vi "Dashboard Main.vi"() -> ()   [LabVIEW 2019]
uses:
  <vilib>/Rock Robotics/WPI/Solenoid/WPI_SolenoidValue.ctl
  <vilib>/Utility/miscctls.llb/LVRowAndColumnTypeDef.ctl
  <vilib>/event_ctls.llb/eventvkey.ctl
  <vilib>/Rock Robotics/Network Tables/NT Read Boolean.vi
  <vilib>/Rock Robotics/Network Tables/NT Write String Array.vi
  <vilib>/Rock Robotics/WPI/Dashboard/WPI_DashboardLogging Global.vi
  <vilib>/Rock Robotics/Network Tables/NT Write Boolean.vi
panel:
  out "Co-Pilot":string="Copilot:\n-LT(0.5 or higher): Intake stow/ deploy toggle\n-RX: Manual Turret Control\n-D-Pad Vertical: Manual Magazine\n-D-Pad Horizontal: Transverse\nMenu: Control panel Pneumatic toggle\nSelect: Elevator Brake\n-LX: Manual Climb Pivot\n-LY: Manual Climb Elevator\n-LB: Automatic climb balancing\n-RB: Toggle Auto_Targeting"
  out "Pilot":string="Pilot\n-LY: Drive Forward\n-RX: Drive Turn\n-Rumble if flywheel spun up and locked on & balls\n-LT(0.5 or more): Intake\n-RT(0.5 or more): Fire and Flywheel spin up\n-RB: control panel manual control \n-LB: Outtake"
  out "appended array":dbl[][](array[numeric])
  in  "TCP":refnum<k5>
  out "Robot IP":string="0.0.0.0"
  out "Image Message":string="Timeout in Camera Communications"
  in  "Dashboard Tab":T1(tab)=enum."Operation"
  in  "Select Auto":string(combo)="Select Autonomous ..."
  out "NT Connection":bool
  out "JS1 Z":dbl(slide) scale=-1.0..1.0 scale format="%#_2e"
  out "JS1 Graph":cluster{"X":dbl, "Y":dbl}[](graph)
  out "JS1 Buttons":T2
  out "JS2 Z":dbl(slide) scale=-1.0..1.0 scale format="%#_2e"
  out "JS2 Graph":cluster{"X":dbl, "Y":dbl}[](graph)
  out "JS2 Buttons":T2
  out "Mode":T3(ring)=enum."Disconnected"
  out "Right Camera Perf":cluster{"Bandwidth (Mbps)":dbl, "FPS":dbl}
  out "Camera Image Right":T4(plugin-control)
  in  "Rec Mode":enum32{"Stop", "Record", "Playback"}(radio)
  in  "Camera Name Right":string(combo)="No Camera Selection"
  in  "Camera Settings Right":T5={"Frame Rate"=15, "Compression"=30, "Size"=1, "DB Camera Config"=FALSE} {"Frame Rate" scale=1.0..30.0; "Compression" scale=100.0..-1.0; "Size" items=["640x480", "320x240", "160x120"]}
  in  "DB/String 9":string
  in  "DB/String 8":string
  in  "DB/String 7":string
  in  "DB/String 6":string
  in  "DB/String 5":string
  in  "DB/String 4":string
  in  "DB/String 3":string
  in  "DB/String 2":string
  in  "DB/String 1":string
  in  "DB/String 0":string
  in  "DB/Slider 0":dbl(slide) scale=0.0..5.0
  in  "DB/Slider 1":dbl(slide) scale=0.0..5.0
  in  "DB/Slider 2":dbl(slide) scale=0.0..5.0
  in  "DB/Slider 3":dbl(slide) scale=0.0..5.0
  out "DB/LED 3":bool
  out "DB/LED 2":bool
  out "DB/LED 1":bool
  out "DB/LED 0":bool
  in  "DB/Button 3":bool
  in  "DB/Button 2":bool
  in  "DB/Button 1":bool
  in  "DB/Button 0":bool caption="New Name"
  in  "Test Slider":dbl(slide) scale=0.0..100.0 scale format="%#_3g"
  in  "On/Off":bool caption="Solenoid"
  in  "Test Name":u16(ring) items=["Select the test to run..."]
  in  "Test Tree":string(tree)
  in  "Motor":cluster{"Value":dbl, "Enable":bool} {"Value" scale=-1.0..1.0 scale format="%#_3g"}
  out "Progress":T6 {"Test Progress" scale=0.0..100.0}
  in  "Rev/Fwd":cluster{"Forward":bool, "Reverse":bool}
  in  "Test Ring":u16(ring) items=["Monochrome", "Color"]
  out "Cmd Status":string
  in  "Execute Command":bool
  in  "Command Params":string[][](table)
  in  "Command Selection":i32(listbox)
  in  "CheckList":i32(listbox)
  in  "Color_Sensor_Values":enum32{"Page 1"}(tab)
  out "Match_Confidence":dbl
  out "Current_B":dbl
  out "Current_G":dbl
  out "Current_R":dbl
  out "Matched_Color_Name":string="No_Value"
  out "Control_Panel":enum32{"Controls"}(tab)
  in  "time_to_run":dbl
  in  "Spinwheel_Throttle":dbl
  in  "Red_B":dbl
  in  "Red_G":dbl
  in  "Red_R":dbl
  in  "Yellow_R":dbl
  in  "Yellow_G":dbl
  in  "Yellow_B":dbl
  in  "Blue_B":dbl
  in  "Blue_G":dbl
  in  "Blue_R":dbl
  in  "Green_R":dbl
  in  "Green_G":dbl
  in  "Green_B":dbl
  out "Magazine":enum32{"Controls"}(tab)
  in  "Max_Magazine_Speed":dbl=1050.0
  in  "Unjam_Speed":dbl
  in  "Firing_Speed":dbl=1.0
  in  "Loading_Speed":dbl=1.0
  in  "Bottom_IR_Theshold":dbl=1.0
  in  "Bottom_Middle_IR_Threshold":dbl=1.5
  in  "Top_Middle_IR_Threshold":dbl=2.0
  in  "Top_IR_Threshold":dbl=1.0
  out "Drive":enum32{"Controls"}(tab)
  in  "Drive_IMU_Yaw":dbl
  in  "Left_P":dbl=1.0
  in  "Left_I":dbl
  in  "Left_D":dbl
  in  "Left_F":dbl
  in  "Right_P":dbl=1.0
  in  "Right_I":dbl
  in  "Right_D":dbl
  in  "Right_F":dbl
  out "Flywheel":enum32{"Controls"}(tab)
  in  "Flywheel_F":dbl=0.0001
  in  "Flywheel_D":dbl
  in  "Flywheel_I":dbl
  in  "Flywheel_P":dbl=0.0001
  out "Turret":enum32{"Controls"}(tab)
  in  "Turret_D":dbl
  in  "Turret_I":dbl=1e-05
  in  "Turret_P":dbl=0.05
  in  "Turret_Upper_Limit":dbl=65.0
  in  "Turret_Lower_Limit":dbl=-90.0
  out "Climb":enum32{"Controls"}(tab)
  out "Intake":enum32{"Controls"}(tab)
  in  "Intake_Speed":dbl=0.7
  in  "extend_delay(ms)":dbl=1000.0
  in  "retract_delay(ms)":dbl=1000.0
  in  "Hopper Input":T7=enum."Reverse"
  in  "Intake Input":T7=enum."Reverse"
  out "No-Op Signal From Robot":bool
  out "Bottom_Middle_IR":bool
  out "Flywheel_Spun_Up":bool
  in  "Auto Selector":string(combo)="No-Op"
  out "Top_IR":bool
  out "Bottom_IR":bool
  out "Top_Middle_IR":bool
  out "Drive_IMU_Yaw":dbl
  out "Climb_IMU_Yaw":dbl
  out "Turret_Relative_Position":dbl
  out "Climb_Bottom_Limit":bool
  out "Climb_Top_Limit":bool
  out "Zero_Turret_Spin":bool
  out "Elevator_Right_Position(Native)":dbl
  out "Elevator_Left_Position(Native)":dbl
  out "Climb_Pivot_Position":dbl
  out "Right_Drive_Position":dbl
  out "Left_Drive_Position":dbl
  out "Control_Panel_Velocity(RPM)":dbl
  out "Control_Panel_Position":dbl
  out "Turret_Velocity(RPM)":dbl
  out "Turret_Absolute_Position":dbl
  out "Magazine_Velocity(RPM)":dbl
  out "Magazine_Position":dbl
  out "Flywheel_Right_Velocity":dbl
  out "Flywheel_Left_Velocity":dbl
  out "Right_Drive_Velocity(RPM)":dbl
  out "Left_Drive_Velocity(RPM)":dbl
  out "Climbing Active":bool
  out "Targetting_Active":bool
  out "Ball Serialized":bool
  out "Match Color Game Data (Stage 3)":string="No_Value"
  out "Camera Image":T4(plugin-control)
  in  "Camera Name":string(combo)="No Camera Selection"
  in  "Camera Settings":T5={"Frame Rate"=15, "Compression"=30, "Size"=1, "DB Camera Config"=FALSE} {"Frame Rate" scale=1.0..30.0; "Compression" scale=100.0..-1.0; "Size" items=["640x480", "320x240", "160x120"]}
  out "Camera Perf":string="                          "
  out "Tree":string(tree)
  out "Background":bool
  # "Joysticks"
  # "Drive Motors"
  # "Front"
  # "Right"
  # "Left"
  # "Back"
  # "HW"
  # "This tab is a great place for autonomous settings and robot-specific values.\nPlace controls and indicators inside this tab and match name to\nDashboard Variables on robot. You can also delete this comment."
  # "HW"
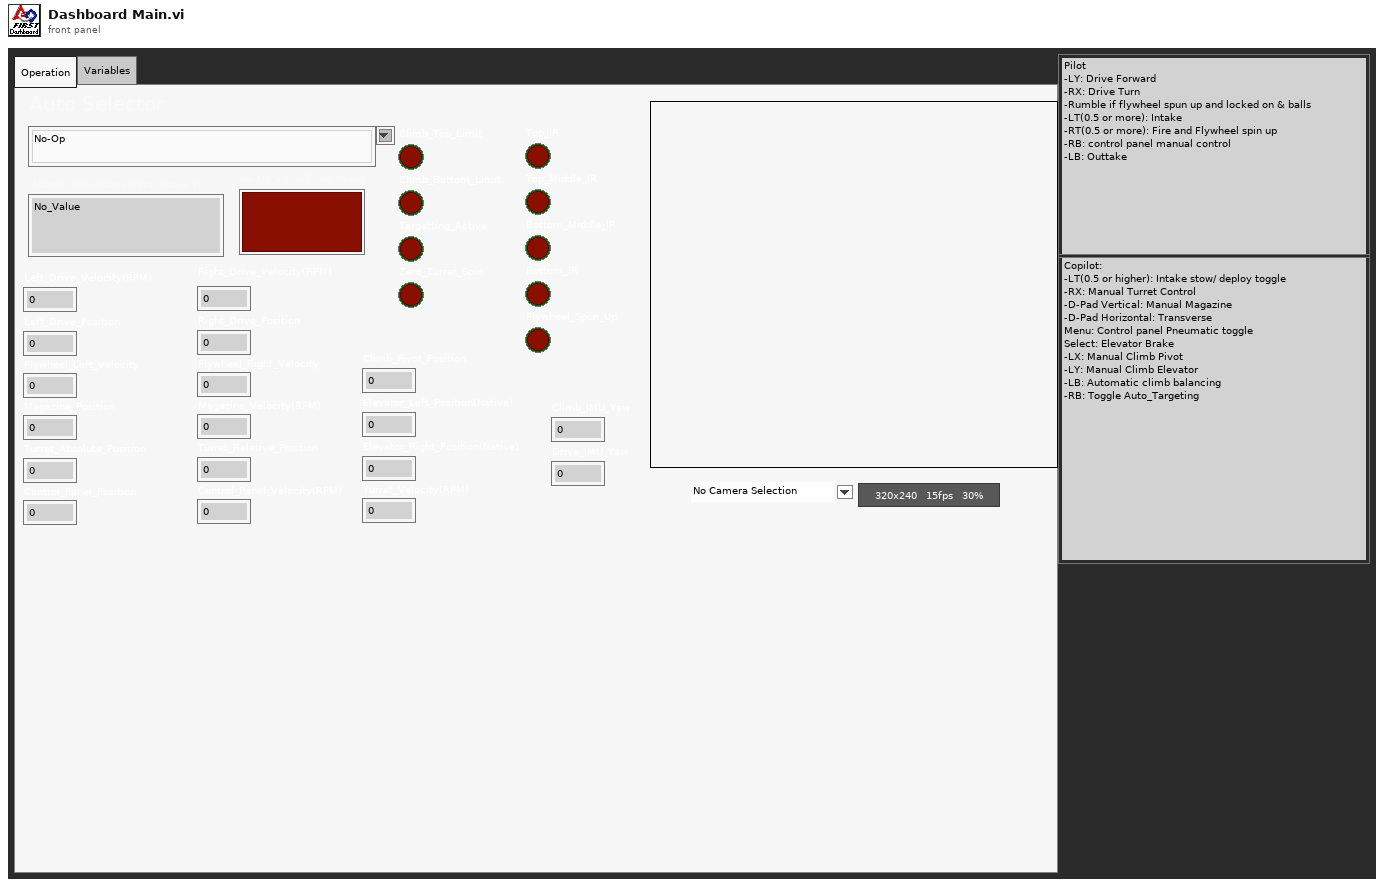
[diagram p1: front panel]
types:
  T1 = enum32{"Drive", "Camera", "Basic", "Custom", "Test", "Commands", "Checklist", "Calibration", "Operation", "Auto", "Variables"}
  T2 = cluster{bool, bool, bool, bool, bool, bool, bool, bool, bool, bool, bool, bool}
  T3 = enum8{"Tele-Op Disabled", "Tele-Op Enabled", "Auto Disabled", "Auto Enabled", "Test Disabled", "Test Enabled", "Disconnected", "No Code", "E-Stop"}
  T4 = typedef "IMAQ Image.ctl" = refnum<image>
  T5 = cluster{"Frame Rate":i32, "Compression":i32, "Size":u16, "DB Camera Config":bool}
  T6 = cluster{"Test Progress":u8, "Test Progress Text":string}
  T7 = typedef "WPI_SolenoidValue.ctl" = enum16{"Off", "On", "Forward", "Reverse"}
  T8 = cluster{"Save Path":path, "Interval (s)":dbl, "Keep":i32}
  T9 = enum32{"Drive", "Camera", "Basic", "Custom", "Test", "Commands", "Checklist", "Variables"}
  T10 = typedef "Image Type" = u32
  T11 = cluster{"IDs":cluster{"RPC field ID":u16, "Unique ID":u16}, "String":string}
  T12 = cluster{"Camera Image":refnum<vi>, "Dashboard Tab":refnum<vi>, "Background":refnum<vi>, "Rec Mode":refnum<vi>, "Test Slider":refnum<vi>, "On/Off ":refnum<vi>, "Test Ring":refnum<vi>, "Rev/Fwd":refnum<vi>, "Test Name":refnum<vi>, "Motor":refnum<vi>, "Progress":refnum<vi>, "CheckList":refnum<vi>, "Tree":refnum<vi>, "Test Tree":refnum<vi>, "Command Params":refnum<vi>, "Command Selection":refnum<vi>, "Execute Command":refnum<vi>, "Cmd Status":refnum<vi>, "Camera Settings":refnum<vi>, "Camera Name":refnum<vi>, "Camera Perf":refnum<vi>, "Camera Settings Right":refnum<vi>, "Camera Name Right":refnum<vi>, "Camera Image Right":refnum<vi>}
  T13 = cluster{"Error Strings":string, "Disable Counts":cluster{u16, u16}, "Rail Faults":cluster{u16, u16, u16}, "Robot IP":string, "DB Mode":u8, "Event Info":cluster{"Name":string, "Type":u8, "Number":u16, "Replay":u8}}
  T14 = cluster{"Storage":cluster{"Disk Free":u64, "RAM Block":u32, "RAM free":u32}, "CPU Utilization":cluster{"CPU % ISR":sgl, "CPU % Time Crit":sgl, "CPU % Timed Str":sgl, "CPU % High":sgl, "CPU % Above":sgl, "CPU % Normal":sgl, "CPU % Low":sgl}, "CAN":cluster{"% Bus Utilization":sgl, "Bus Off Cnt":u32, "TX_FIFO Full Cnt":u32, "Receive Error Cnt":u8, "Transmit Error Cnt":u8}, "HID":cluster{"HID Outputs":u32, "Rumble Low":u16, "Rumble High":u16}[]}
  T15 = cluster{"Status bits":cluster{"Test Mode":bool, "Autonomous":bool, "Enabled":bool, "Code Start":bool, "Brownout":bool, "Reserved 2":bool, "Reserved 3":bool, "E-Stop":bool}, "Code Trace":cluster{"Disabled":bool, "TeleOp":bool, "Auto":bool, "Test":bool}, "Controller Type":enum16{"unknown", "cRIO", "roboRio"}, "Code?":enum16{"unknown", "noCode", "code"}, "Battery V":dbl}
  T16 = cluster{"Control Bits":cluster{"TestMode":bool, "Autonomous":bool, "Enabled":bool, "FMS Present":bool, bool, bool, bool, "E-Stop":bool}, "Team Station ":u8, "Countdown":sgl, "Joystick Values":cluster{"Axes":dbl[], "Buttons":bool[], "POVs":i16[]}[]}
  T17 = cluster{"Axes":dbl[], "Buttons":bool[], "POVs":i16[]}[]
  T18 = cluster{"Axes":dbl[], "Buttons":bool[], "POVs":i16[]}
  T19 = cluster{"Buttons[0]":bool, "Buttons[1]":bool, "Buttons[2]":bool, "Buttons[3]":bool, "Buttons[4]":bool, "Buttons[5]":bool, "Buttons[6]":bool, "Buttons[7]":bool, "Buttons[8]":bool, "Buttons[9]":bool, "Buttons[10]":bool, "Buttons[11]":bool}
  T20 = cluster{"Global Rectangle":i32[], "Contours":cluster{"Contour Type":u32, "ROI Type":u32, "Points":i32[]}[]}
  T21 = cluster{"Camera Name":string, string, "Saved DB Images Info":cluster{"Save Path":path, "Interval (s)":dbl, "Keep":i32}}
  T22 = cluster{"Camera Name Right":string, string, "Saved DB Images Info":cluster{"Save Path":path, "Interval (s)":dbl, "Keep":i32}}
  T23 = cluster{"Operation":enum16{"Update", "Clear"}, "Color Box":u32}[]
  T24 = typedef "eventvkey.ctl" = enum16{"ASCII", "Enter", "Return", "Shift", "Ctrl", "Alt", "Cmd", "Opt", "Caps", "NumLock", "Clear", "Break", "Up", "Down", "Left", "Right", "Insert", "Delete", "Home", "End", "PageUp", "PageDown", "Escape", "Help", "Pause", "ScrollLock", "F1", "F2", "F3", "F4", "F5", "F6", "F7", "F8", "F9", "F10", "F11", "F12", "F13", "F14", "F15", "F16", "F17", "F18", "F19", "F20", "F21", "F22", "F23", "F24", "Play", "VolumeUp", "VolumeDown", "Mute", "Two Byte Char"}
  T25 = cluster{"Image Size":bool, "Image Type":bool, "Pixel Value":bool, "ROI Information":bool, "Zoom Factor":bool}
  T26 = cluster{"Operation":enum16{"Update", "Clear"}, "Color Box":u32}
  T27 = typedef "LVRowAndColumnTypeDef.ctl" = cluster{"Row":i32, "Column":i32}
  T28 = cluster{"Shift":bool, "Ctrl":bool, "Alt":bool, "Cmd":bool, "Opt":bool}
  T29 = enum32{"Drive", "Camera", "Basic", "Custom", "Test", "Commands", "Checklist", "Variables", "Calibration"}
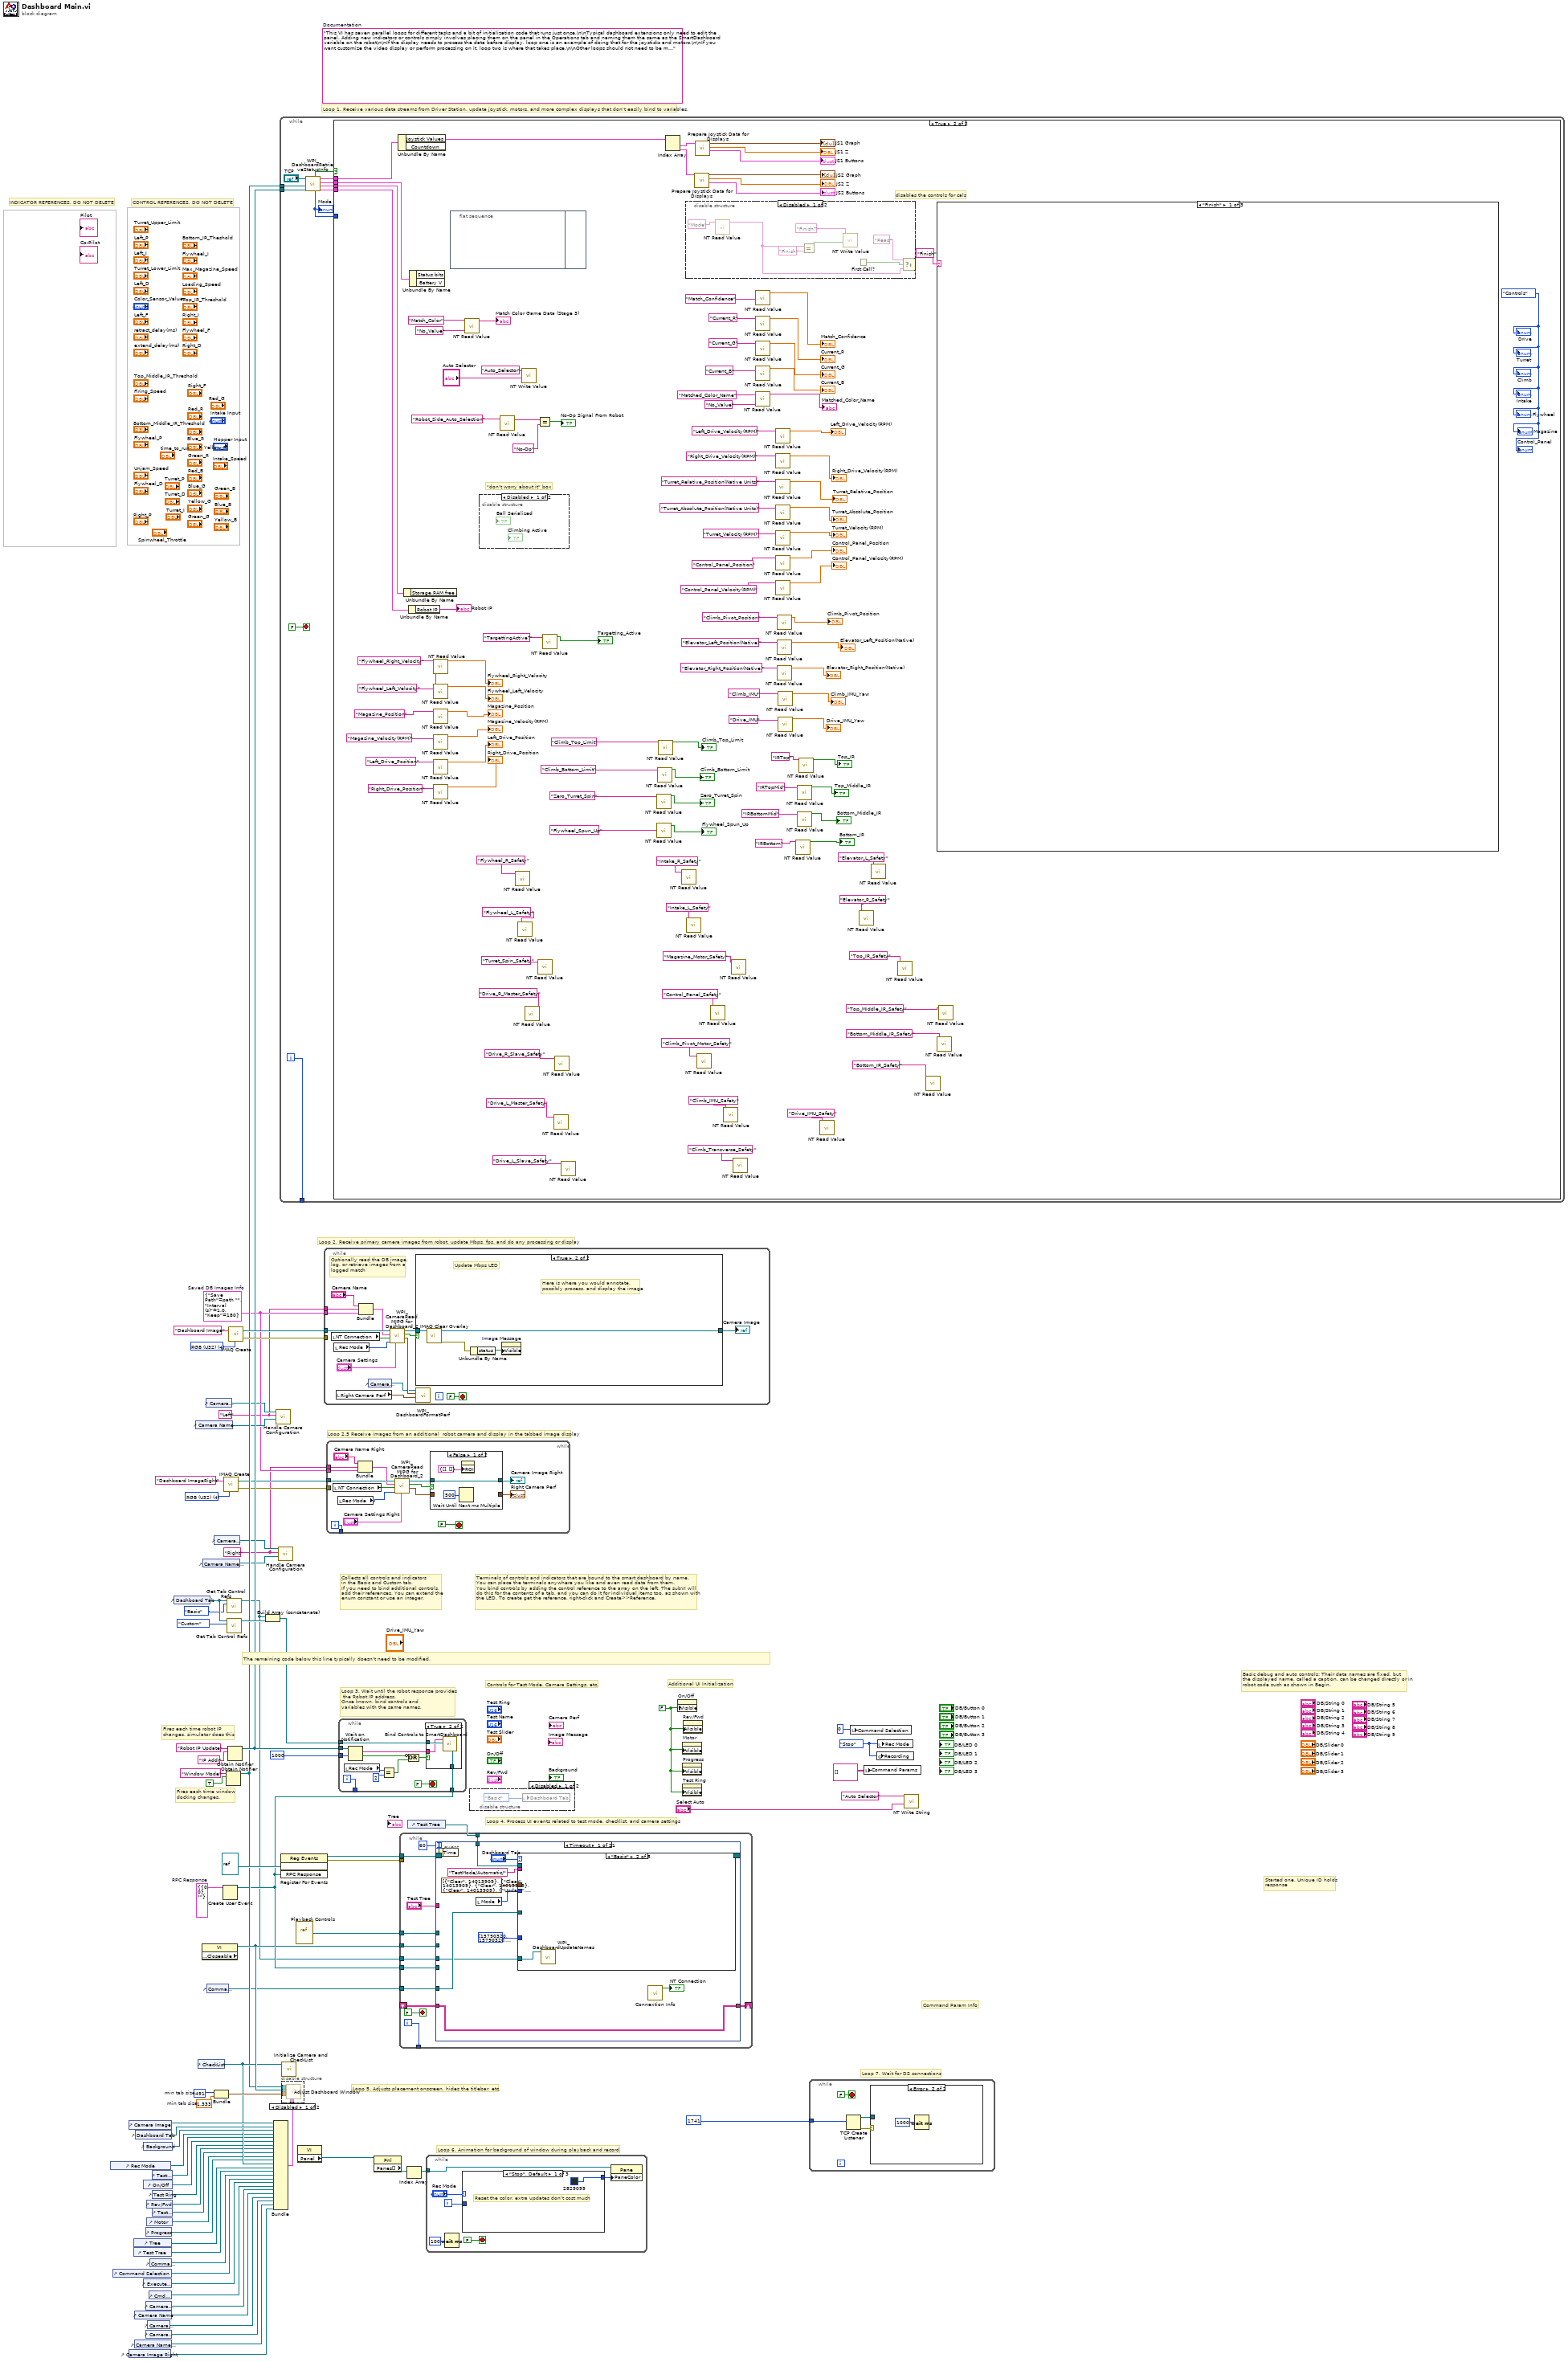
[diagram p0: block diagram]
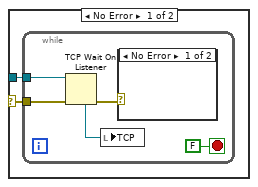
[diagram p5: hidden frame]
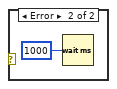
[diagram p6: hidden frame]
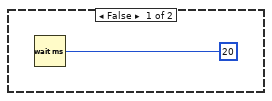
[diagram p7: hidden frame]
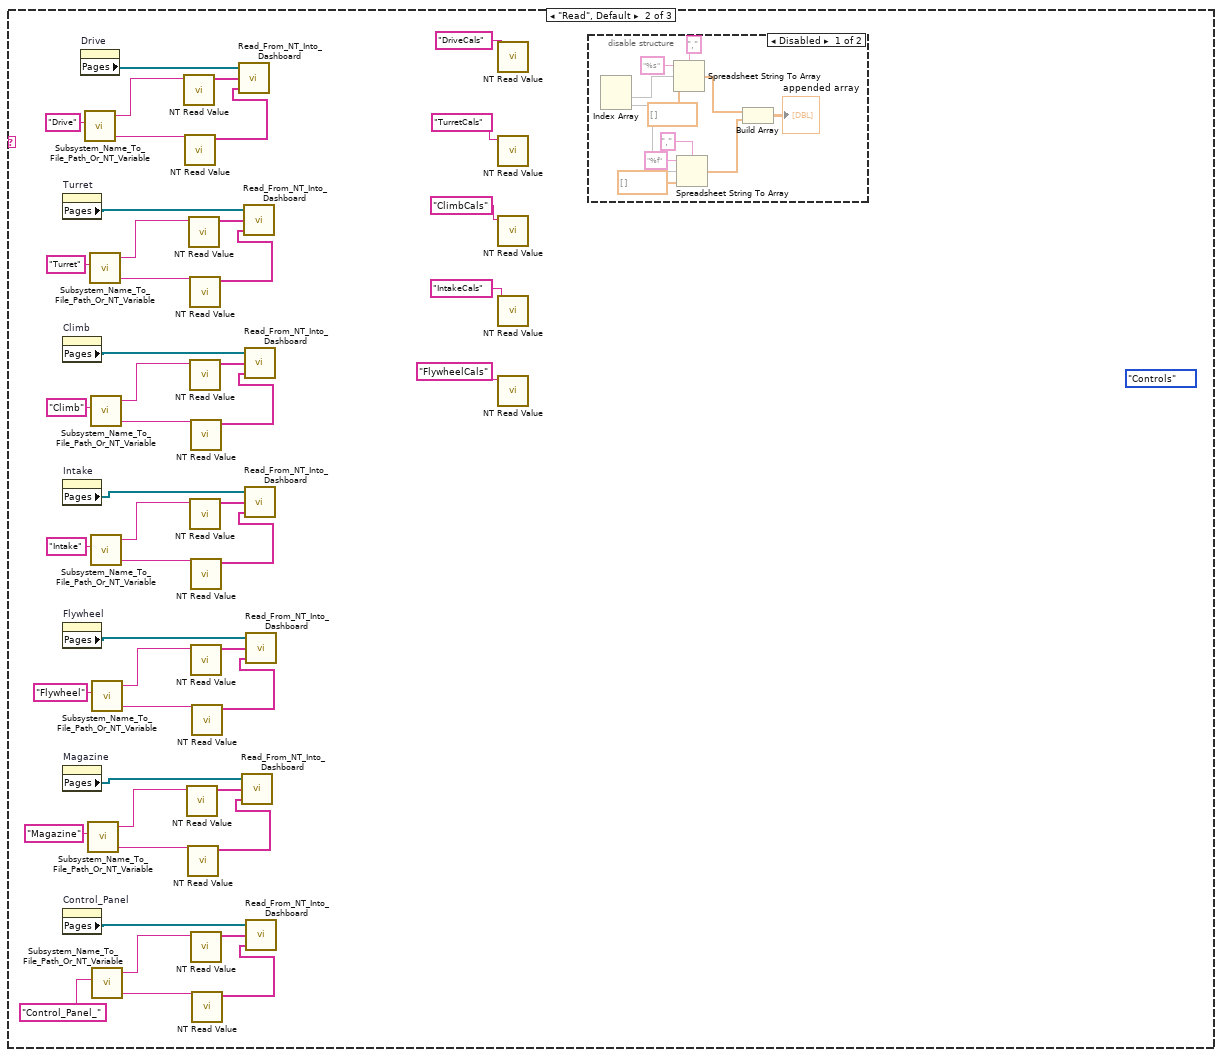
[diagram p10: hidden frame]
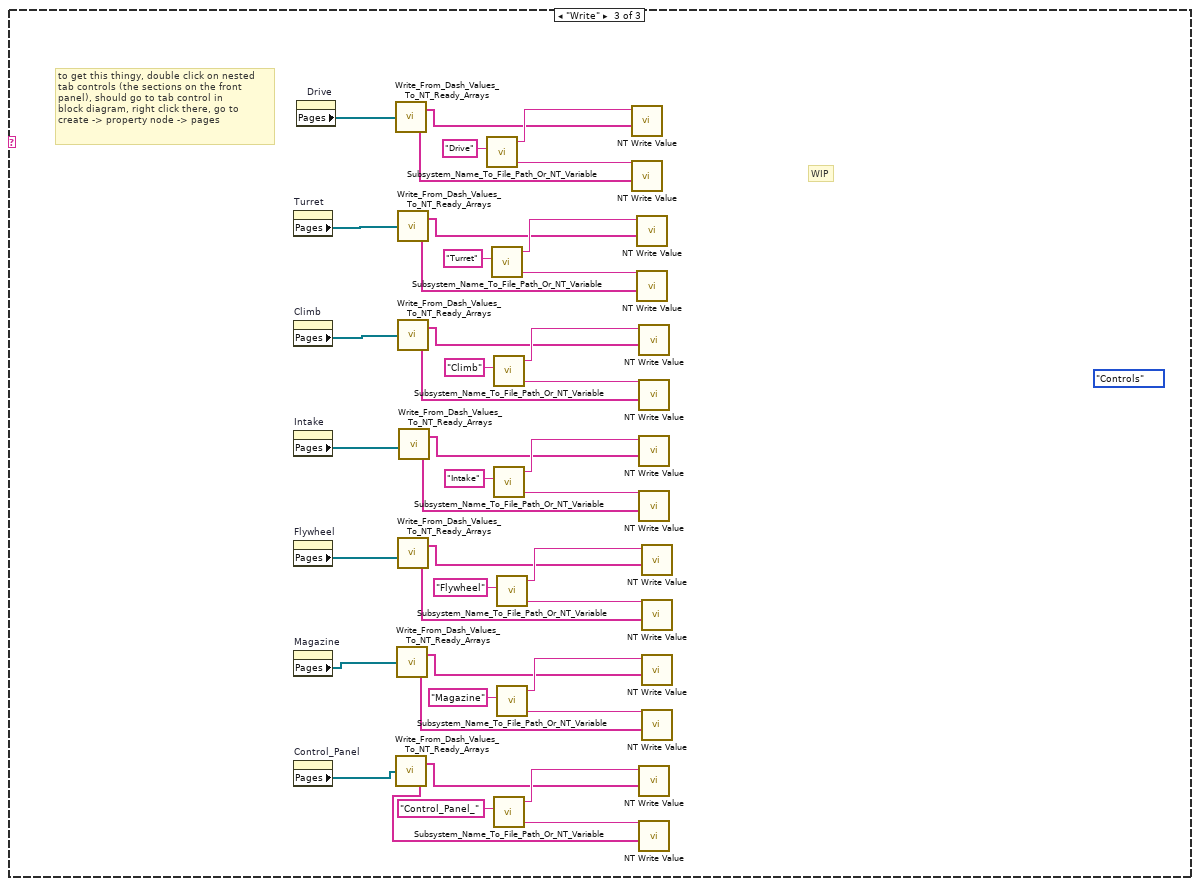
[diagram p12: hidden frame]
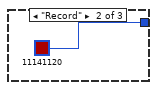
[diagram p13: hidden frame]
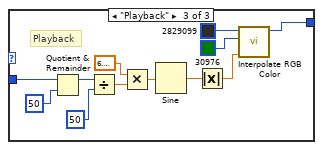
[diagram p14: hidden frame]
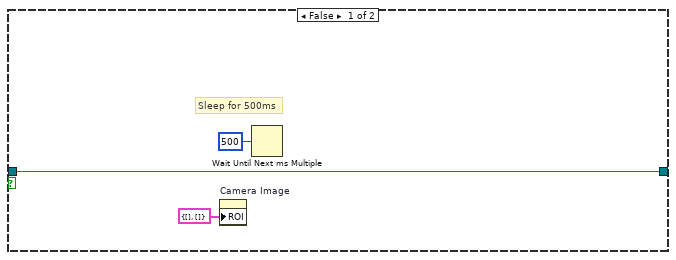
[diagram p16: hidden frame]
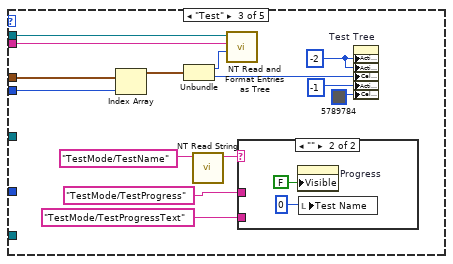
[diagram p18: hidden frame]
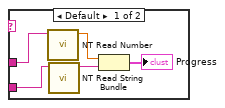
[diagram p19: hidden frame]
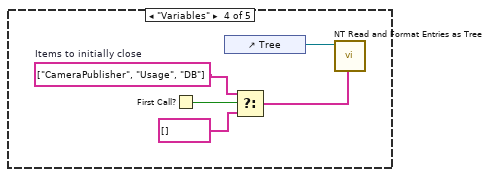
[diagram p20: hidden frame]
diagram:
  w3 = T8 {"Save Path"=path "", "Interval (s)"=1.0, "Keep"=180}  # Saved DB Images Info
  w2 = "Right"
  w1 = "Left"
  w13 = T10 4 items=["Grayscale (U8)", "Grayscale (I16)", "Grayscale (SGL)", "Complex (CSG)", "RGB (U32)", "HSL (U32)", "RGB (U64)"] ("Image Type")
  w29 = T11 {"IDs"={"RPC field ID"=0, "Unique ID"=0}, "String"=""}  # RPC Response
  w51 = 491  # min tab size
  w50 = 1.333  # min tab size
  w58 = enum32{"Stop", "Record", "Playback"}."Stop" ("Rec Mode")
  w35 = FALSE ("Visible")
  (unwired) "This VI has seven parallel loops for different tasks and a bit of initialization code that runs just once.\n\nTypical dashboard extensions only need to edit the panel. Adding new indicators or controls simply involves placing them on the panel in the Operations tab and naming them the same as the SmartDashboard variable on the robot\n\nIf the display needs to process the data before display, loop one is an example of doing that for the joysticks and motors.\n\nIf you want customize the video display or perform processing on it, loop two is where that takes place.\n\nOther loops should not need to be modified. They are pretty standard, and document the task they perform."  # Documentation
  w75 = T10 4 items=["Grayscale (U8)", "Grayscale (I16)", "Grayscale (SGL)", "Complex (CSG)", "RGB (U32)", "HSL (U32)", "RGB (U64)"] ("Image Type")
  # "INDICATOR REFERENCES, DO NOT DELETE"
  # "CONTROL REFERENCES, DO NOT DELETE"
  # "Loop 2.5 Receive images from an additional  robot camera and display in the tabbed image display"
  # "Command Param Info"
  # "Started one, Unique ID holds\nresponse"
  # "Loop 7. Wait for DS connections"
  # "Basic debug and auto controls: Their data names are fixed, but\nthe displayed name, called a caption, can be changed directly or in\nrobot code such as shown in Begin."
  # "Controls for Test Mode, Camera Settings, etc."
  # "Additional UI Initialization"
  # "Loop 6. Animation for background of window during playback and record"
  # "Fires each time robot IP\nchanges, simulator does this"
  # "Fires each time window\ndocking changes."
  # "Collects all controls and indicators\nin the Basic and Custom tab.\nIf you need to bind additional controls,\nadd their references. You can extend the\nenum constant or use an integer."
  # "The remaining code below this line typically doesn't need to be modified."
  # "Loop 4. Process UI events related to test mode, checklist, and camera settings"
  # "Terminals of controls and indicators that are bound to the smart dashboard by name.\nYou can place the terminals anywhere you like and even read data from them.\nYou bind controls by adding the control reference to the array on the left. The subVI will\ndo this for the contents of a tab, and you can do it for individual items too, as shown with\nthe LED. To create get the reference, right-click and Create>>Reference."
  # "Loop 3. Wait until the robot response provides\n the Robot IP address.\nOnce known, bind controls and\nvariables with the same names."
  # "Loop 5. Adjusts placement onscreen, hides the titlebar, etc."
  # "Loop 1. Receive various data streams from Driver Station, update joystick, motors, and more complex displays that don't easily bind to variables."
  # "Loop 2. Receive primary camera images from robot, update Mbps, fps, and do any processing or display"
  n1 = control-ref of="Rec Mode"() -> (w41:refnum<vi>)
  n2 = control-ref of="Command Selection"() -> (w28:refnum<vi>)
  n3 = control-ref of="Camera Image Right"() -> (w6:refnum<vi>)
  n4 = control-ref of="Camera Image"() -> (w53:refnum<vi>)
  n5 = control-ref of="Tree"() -> (w45:refnum<vi>)
  n6 = control-ref of="Test Tree"() -> (w44:refnum<vi>)
  n7 = control-ref of="Camera Name"() -> (w19:refnum<vi>)
  n8 = control-ref of="Camera Name Right"() -> (w7:refnum<vi>)
  n9 = control-ref of="Dashboard Tab"() -> (w52:refnum<vi>)
  n10 = control-ref of="Execute Command"() -> (w30:refnum<vi>)
  n11 = control-ref of="Background"() -> (w48:refnum<vi>)
  n12 = control-ref of="On/Off"() -> (w39:refnum<vi>)
  n13 = control-ref of="Progress"() -> (w36:refnum<vi>)
  n14 = control-ref of="Camera Settings"() -> (w20:refnum<vi>)
  n15 = control-ref of="Camera Settings Right"() -> (w8:refnum<vi>)
  n16 = control-ref of="Rev/Fwd"() -> (w37:refnum<vi>)
  n17 = control-ref of="Motor"() -> (w42:refnum<vi>)
  n18 = control-ref of="Camera Perf"() -> (w18:refnum<vi>)
  n19 = control-ref of="Cmd Status"() -> (w24:refnum<vi>)
  n20 = control-ref of="Command Params"() -> (w31:refnum<vi>)
  n21 = control-ref of="Test Slider"() -> (w40:refnum<vi>)
  n22 = control-ref of="Test Ring"() -> (w38:refnum<vi>)
  n23 = control-ref of="Test Name"() -> (w43:refnum<vi>)
  n24 = control-ref of="Dashboard Tab"() -> (w56:refnum<vi>)
  n25 = control-ref of="Camera Name"() -> (w21:refnum<vi>)
  n26 = control-ref of="CheckList"() -> (w46:refnum<vi>)
  n27 = property class="VI" props=["Front Panel.Closeable"]() -> (reference out=w57:refnum<vi>)  [unwired: 2 in, 2 out]
  n28 = control-ref of="Camera Name Right"() -> (w9:refnum<vi>)
  n29 = control-ref of="Camera Settings"() -> (w22:refnum<vi>)
  n30 = control-ref of="Command Params"() -> (w23:refnum<vi>)
  n31 = control-ref of="Camera Settings Right"() -> (w10:refnum<vi>)
  n32 = Bundle("min tab size"=w51, "min tab size"=w50) -> (w49:cluster{"min tab size":i32, "min tab size":dbl})  [unwired: 1 in]
  n33 = Create User Event(user event datatype=w29) -> (user event=w25:refnum<user-event>)  [unwired: 1 in, 1 out]
  n34 = call "IMAQ Create"("Image Name"="Dashboard ImageRight", "Image Type"=w13) -> ("New Image"=w12:T4, "error out"=w11:errorcluster)  [unwired: 2 in, 1 out]
  n35 = Obtain Notifier(name (unnamed)="Window Mode", notification data type=TRUE) -> (notifier out=w33:refnum<notifier>)  [unwired: 2 in, 2 out]
  n36 = call <vilib>:"Get Tab Control Refs.vi"("Page Index"=T9."Basic" ("Dashboard Tab"), "TabControl in"=w56) -> ("ControlsOnPage"=w17:refnum<vi>[])  [unwired: 9 in]
  n37 = call <vilib>:"Get Tab Control Refs.vi"("Page Index"=T9."Custom" ("Dashboard Tab"), "TabControl in"=w56) -> ("ControlsOnPage"=w55:refnum<vi>[])  [unwired: 9 in]
  n38 = Obtain Notifier(name (unnamed)="Robot IP Update", notification data type="IP Addr" ("name (unnamed)")) -> (notifier out=w34:refnum<notifier>)  [unwired: 2 in, 2 out]
  n39 = call "IMAQ Create"("Image Name"="Dashboard Image", "Image Type"=w75) -> ("New Image"=w73:T4, "error out"=w72:errorcluster)  [unwired: 2 in, 1 out]
  n40 = Build Array (concatenate)(w17, w55) -> (w54:refnum<vi>[])
  n41 = Bundle("Camera Image"=w53, "Dashboard Tab"=w52, "Background"=w48, "Rec Mode"=w41, "Test Slider"=w40, "On/Off"=w39, "Test Ring"=w38, "Rev/Fwd"=w37, "Test Name"=w43, "Motor"=w42, "Progress"=w36, "CheckList"=w46, "Tree"=w45, "Test Tree"=w44, "Command Params"=w31, "Command Selection"=w28, "Execute Command"=w30, "Cmd Status"=w24, "Camera Settings"=w20, "Camera Name"=w19, "Camera Perf"=w18, "Camera Settings Right"=w8, "Camera Name Right"=w7, "Camera Image Right"=w6) -> (w47:T12)  [unwired: 1 in]
  n42 = call "Handle Camera Configuration.vi"("CameraNameRef"=w21, "Display Name"=w1, "ClusterRef"=w22) -> ()  [unwired: 9 in]
  n43 = call "Handle Camera Configuration.vi"("CameraNameRef"=w9, "Display Name"=w2, "ClusterRef"=w10) -> ()  [unwired: 9 in]
  n44 = while {
    tunnel: [w85] -> _
    tunnel: w34 -> [w80]
    tunnel: w33 -> [w77]
    i -> [w85]
    stop <- FALSE stop-if-true
    n45 = call <vilib>:"WPI_DashboardRetrieveStatusInfo.vi"("Binding Refnum"=w80, "Window Mode Notifier"=w77, "TCP Cnx"="TCP") -> ("Power and Errors"=w81:T13, "Robot Metrics"=w83:T14, "Status Info"=w84:T15, "Control Info"=w82:T16, "Robot Mode"=w79:T3, "Process?"=w76:bool)  [unwired: 3 in]
    "Mode" <- w79
    n46 = case shown="True" w76 {
      tunnel: w84 -> [_ w198]
      tunnel: w83 -> [_ w197]
      tunnel: w82 -> [_ w196]
      tunnel: w81 -> [_ w195]
      tunnel: w79 -> [_ _]
      frame False {
        n47 = Wait (ms)(milliseconds to wait=u32 20) -> ()  [unwired: 1 out]
      }
      frame True {
        w181 = enum32{"Controls", "Indicators"}."Controls" ("Climb")
        # "disables the controls for cals"
        # "\"don't worry about it\" box"
        n48 = Unbundle By Name(w196) -> ("Joystick Values"=w194:T17)  [unwired: 1 out]
        n49 = Unbundle By Name(w197) -> ()  [unwired: 1 out]
        n50 = Unbundle By Name(w195) -> ("Robot IP"=→"Robot IP":string)
        n51 = Unbundle By Name(w198) -> ()  [unwired: 2 out]
        n52 = call-poly <vilib>:"NT Read Value.vi"("Name"="Flywheel_Left_Velocity") -> ("Numeric"=→"Flywheel_Right_Velocity":dbl)  [unwired: 9 in, 1 out]
        n53 = call-poly <vilib>:"NT Read Value.vi"("Name"="Flywheel_Right_Velocity") -> ("Numeric"=→"Flywheel_Left_Velocity":dbl)  [unwired: 9 in, 1 out]
        n54 = call-poly <vilib>:"NT Read Value.vi"("Name"="Magazine_Position") -> ("Numeric"=→"Magazine_Position":dbl)  [unwired: 9 in, 1 out]
        n55 = call-poly <vilib>:"NT Read Value.vi"("Name"="Magazine_Velocity(RPM)") -> ("Numeric"=→"Magazine_Velocity(RPM)":dbl)  [unwired: 9 in, 1 out]
        n56 = call-poly <vilib>:"NT Read Value.vi"("Name"="Left_Drive_Position") -> ("Numeric"=→"Left_Drive_Position":dbl)  [unwired: 9 in, 1 out]
        n57 = call-poly <vilib>:"NT Read Value.vi"("Name"="Right_Drive_Position") -> ("Numeric"=→"Right_Drive_Position":dbl)  [unwired: 9 in, 1 out]
        n58 = flat-sequence {
          frame #0 {
          }
          frame #1 {
          }
        }
        n59 = call-poly <vilib>:"NT Read Value.vi"("Default Value"="No_Value", "Name"="Match_Color") -> ("String"=→"Match Color Game Data (Stage 3)":string)  [unwired: 8 in, 1 out]
        n60 = disable-structure shown="Disabled" {
          frame Disabled {
          }
          frame Enabled {
          }
        }
        n61 = call-poly <vilib>:"NT Read Value.vi"("Name"="Robot_Side_Auto_Selection") -> ("String"=w90:string)  [unwired: 9 in, 1 out]
        n62 = call-poly <vilib>:"NT Read Value.vi"("Name"="Flywheel_R_Safety") -> ()  [unwired: 9 in, 2 out]
        n63 = call-poly <vilib>:"NT Read Value.vi"("Name"="Flywheel_L_Safety") -> ()  [unwired: 9 in, 2 out]
        n64 = call-poly <vilib>:"NT Write Value.vi"("String"="Auto Selector", "Name"="Auto_Selector") -> ()  [unwired: 9 in, 1 out]
        n65 = call-poly <vilib>:"NT Read Value.vi"("Name"="Drive_R_Master_Safety") -> ()  [unwired: 9 in, 2 out]
        n66 = Equal?(x=w90, y="No-Op") -> (x = y?=→"No-Op Signal From Robot":bool)
        n67 = call-poly <vilib>:"NT Read Value.vi"("Name"="Turret_Spin_Safety") -> ()  [unwired: 9 in, 2 out]
        n68 = call-poly <vilib>:"NT Read Value.vi"("Name"="TargettingActive?") -> ("Boolean"=→"Targetting_Active":bool)  [unwired: 9 in, 1 out]
        n69 = call-poly <vilib>:"NT Read Value.vi"("Name"="Drive_L_Master_Safety") -> ()  [unwired: 9 in, 2 out]
        n70 = call-poly <vilib>:"NT Read Value.vi"("Name"="Drive_R_Slave_Safety") -> ()  [unwired: 9 in, 2 out]
        n71 = call-poly <vilib>:"NT Read Value.vi"("Name"="Drive_L_Slave_Safety") -> ()  [unwired: 9 in, 2 out]
        n72 = call-poly <vilib>:"NT Read Value.vi"("Name"="Zero_Turret_Spin") -> ("Boolean"=→"Zero_Turret_Spin":bool)  [unwired: 9 in, 1 out]
        n73 = call-poly <vilib>:"NT Read Value.vi"("Name"="Flywheel_Spun_Up") -> ("Boolean"=→"Flywheel_Spun_Up":bool)  [unwired: 9 in, 1 out]
        n74 = call-poly <vilib>:"NT Read Value.vi"("Name"="Climb_Bottom_Limit") -> ("Boolean"=→"Climb_Bottom_Limit":bool)  [unwired: 9 in, 1 out]
        n75 = call-poly <vilib>:"NT Read Value.vi"("Name"="Climb_Top_Limit") -> ("Boolean"=→"Climb_Top_Limit":bool)  [unwired: 9 in, 1 out]
        n76 = Index Array(array=w194) -> (element #1=w193:T18, element #2=w189:T18)  [unwired: 2 in]
        n77 = call-poly <vilib>:"NT Read Value.vi"("Name"="Intake_R_Safety") -> ()  [unwired: 9 in, 2 out]
        n78 = disable-structure shown="Disabled" {
          frame Disabled {
            n79 = call-poly <vilib>:"NT Read Value.vi"("Name"="Mode") -> ("String"=w199:string)  [unwired: 9 in, 1 out]
            n80 = Equal?(x=w199, y="Finish") -> (x = y?=w203:bool)
            n81 = call-poly <vilib>:"NT Write Value.vi"("Boolean"=w203, "Name"="Finish?") -> ()  [unwired: 9 in, 1 out]
            n82 = First Call?() -> (First Call?: T/F=w201:bool)
            n83 = Select(t="Read" ("f"), s=w201, f=w199) -> ()  [unwired: 1 out]
          }
          frame Enabled {
          }
        }
        n84 = call-poly <vilib>:"NT Read Value.vi"("Name"="Intake_L_Safety") -> ()  [unwired: 9 in, 2 out]
        n85 = call "Prepare Joystick Data for Displays.vi"("Joystick Values"=w189) -> ("Buttons"=→"JS2 Buttons":T19, "Z Axis"=→"JS2 Z":dbl, "Cartesian Data"=→"JS2 Graph":cluster{"X axis":dbl, "X axis":dbl}[])  [unwired: 8 in]
        n86 = call "Prepare Joystick Data for Displays.vi"("Joystick Values"=w193) -> ("Buttons"=→"JS1 Buttons":T19, "Z Axis"=→"JS1 Z":dbl, "Cartesian Data"=→"JS1 Graph":cluster{"X axis":dbl, "X axis":dbl}[])  [unwired: 8 in]
        n87 = call-poly <vilib>:"NT Read Value.vi"("Name"="Climb_Pivot_Motor_Safety") -> ()  [unwired: 9 in, 2 out]
        n88 = call-poly <vilib>:"NT Read Value.vi"("Name"="Control_Panel_Safety") -> ()  [unwired: 9 in, 2 out]
        n89 = call-poly <vilib>:"NT Read Value.vi"("Name"="Climb_IMU_Safety") -> ()  [unwired: 9 in, 2 out]
        n90 = call-poly <vilib>:"NT Read Value.vi"("Name"="Magazine_Motor_Safety") -> ()  [unwired: 9 in, 2 out]
        n91 = call-poly <vilib>:"NT Read Value.vi"("Name"="Climb_Transverse_Safety") -> ()  [unwired: 9 in, 2 out]
        n92 = call-poly <vilib>:"NT Read Value.vi"("Default Value"="No_Value", "Name"="Matched_Color_Name") -> ("String"=→"Matched_Color_Name":string)  [unwired: 8 in, 1 out]
        n93 = call-poly <vilib>:"NT Read Value.vi"("Name"="Match_Confidence") -> ("Numeric"=→"Match_Confidence":dbl)  [unwired: 9 in, 1 out]
        n94 = call-poly <vilib>:"NT Read Value.vi"("Name"="Current_R") -> ("Numeric"=→"Current_R":dbl)  [unwired: 9 in, 1 out]
        n95 = call-poly <vilib>:"NT Read Value.vi"("Name"="Current_G") -> ("Numeric"=→"Current_G":dbl)  [unwired: 9 in, 1 out]
        n96 = call-poly <vilib>:"NT Read Value.vi"("Name"="Current_B") -> ("Numeric"=→"Current_B":dbl)  [unwired: 9 in, 1 out]
        n97 = call-poly <vilib>:"NT Read Value.vi"("Name"="Turret_Relative_Position(Native Units)") -> ("Numeric"=→"Turret_Relative_Position":dbl)  [unwired: 9 in, 1 out]
        n98 = call-poly <vilib>:"NT Read Value.vi"("Name"="Left_Drive_Velocity(RPM)") -> ("Numeric"=→"Left_Drive_Velocity(RPM)":dbl)  [unwired: 9 in, 1 out]
        n99 = call-poly <vilib>:"NT Read Value.vi"("Name"="Right_Drive_Velocity(RPM)") -> ("Numeric"=→"Right_Drive_Velocity(RPM)":dbl)  [unwired: 9 in, 1 out]
        n100 = call-poly <vilib>:"NT Read Value.vi"("Name"="Turret_Absolute_Position(Native Units)") -> ("Numeric"=→"Turret_Absolute_Position":dbl)  [unwired: 9 in, 1 out]
        n101 = call-poly <vilib>:"NT Read Value.vi"("Name"="Turret_Velocity(RPM)") -> ("Numeric"=→"Turret_Velocity(RPM)":dbl)  [unwired: 9 in, 1 out]
        n102 = call-poly <vilib>:"NT Read Value.vi"("Name"="Control_Panel_Position") -> ("Numeric"=→"Control_Panel_Position":dbl)  [unwired: 9 in, 1 out]
        n103 = call-poly <vilib>:"NT Read Value.vi"("Name"="Control_Panel_Velocity(RPM)") -> ("Numeric"=→"Control_Panel_Velocity(RPM)":dbl)  [unwired: 9 in, 1 out]
        n104 = call-poly <vilib>:"NT Read Value.vi"("Name"="Climb_Pivot_Position") -> ("Numeric"=→"Climb_Pivot_Position":dbl)  [unwired: 9 in, 1 out]
        n105 = call-poly <vilib>:"NT Read Value.vi"("Name"="Elevator_Left_Position(Native)") -> ("Numeric"=→"Elevator_Left_Position(Native)":dbl)  [unwired: 9 in, 1 out]
        n106 = call-poly <vilib>:"NT Read Value.vi"("Name"="Elevator_Right_Position(Native)") -> ("Numeric"=→"Elevator_Right_Position(Native)":dbl)  [unwired: 9 in, 1 out]
        n107 = call-poly <vilib>:"NT Read Value.vi"("Name"="Climb_IMU") -> ("Numeric"=→"Climb_IMU_Yaw":dbl)  [unwired: 9 in, 1 out]
        n108 = call-poly <vilib>:"NT Read Value.vi"("Name"="Drive_IMU") -> ("Numeric"=→"Drive_IMU_Yaw":dbl)  [unwired: 9 in, 1 out]
        n109 = call-poly <vilib>:"NT Read Value.vi"("Name"="IRBottom") -> ("Boolean"=→"Bottom_IR":bool)  [unwired: 9 in, 1 out]
        n110 = call-poly <vilib>:"NT Read Value.vi"("Name"="IRTopMid") -> ("Boolean"=→"Top_Middle_IR":bool)  [unwired: 9 in, 1 out]
        n111 = call-poly <vilib>:"NT Read Value.vi"("Name"="IRBottomMid") -> ("Boolean"=→"Bottom_Middle_IR":bool)  [unwired: 9 in, 1 out]
        n112 = call-poly <vilib>:"NT Read Value.vi"("Name"="IRTop") -> ("Boolean"=→"Top_IR":bool)  [unwired: 9 in, 1 out]
        n113 = call-poly <vilib>:"NT Read Value.vi"("Name"="Drive_IMU_Safety") -> ()  [unwired: 9 in, 2 out]
        n114 = call-poly <vilib>:"NT Read Value.vi"("Name"="Elevator_R_Safety") -> ()  [unwired: 9 in, 2 out]
        n115 = call-poly <vilib>:"NT Read Value.vi"("Name"="Elevator_L_Safety") -> ()  [unwired: 9 in, 2 out]
        n116 = call-poly <vilib>:"NT Read Value.vi"("Name"="Top_IR_Safety") -> ()  [unwired: 9 in, 2 out]
        n117 = call-poly <vilib>:"NT Read Value.vi"("Name"="Bottom_IR_Safety") -> ()  [unwired: 9 in, 2 out]
        n118 = call-poly <vilib>:"NT Read Value.vi"("Name"="Bottom_Middle_IR_Safety") -> ()  [unwired: 9 in, 2 out]
        n119 = case shown="\"Finish\"" "Finish" {
          frame "Finish" {
          }
          frame "Read", Default {
            (unwired) enum32{"Controls", "Indicators"}."Controls" ("Climb")
            n120 = property on="Turret" class="TabCtl (strict)"() -> ("Pages"=w211:refnum<vi>[])  [unwired: 2 in, 2 out]
            n121 = property on="Climb" class="TabCtl (strict)"() -> ("Pages"=w210:refnum<vi>[])  [unwired: 2 in, 2 out]
            n122 = property on="Intake" class="TabCtl (strict)"() -> ("Pages"=w209:refnum<vi>[])  [unwired: 2 in, 2 out]
            n123 = property on="Flywheel" class="TabCtl (strict)"() -> ("Pages"=w208:refnum<vi>[])  [unwired: 2 in, 2 out]
            n124 = property on="Magazine" class="TabCtl (strict)"() -> ("Pages"=w207:refnum<vi>[])  [unwired: 2 in, 2 out]
            n125 = property on="Control_Panel" class="TabCtl (strict)"() -> ("Pages"=w206:refnum<vi>[])  [unwired: 2 in, 2 out]
            n126 = property on="Drive" class="TabCtl (strict)"() -> ("Pages"=w247:refnum<vi>[])  [unwired: 2 in, 2 out]
            n127 = call "Subsystem_Name_To_File_Path_Or_NT_Variable.vi"("Enum String Name"="Drive") -> ("Names"=w245:string, "Values"=w244:string)  [unwired: 5 in, 1 out]
            n128 = call "Subsystem_Name_To_File_Path_Or_NT_Variable.vi"("Enum String Name"="Magazine") -> ("Names"=w220:string, "Values"=w219:string)  [unwired: 5 in, 1 out]
            n129 = call "Subsystem_Name_To_File_Path_Or_NT_Variable.vi"("Enum String Name"="Turret") -> ("Names"=w240:string, "Values"=w239:string)  [unwired: 5 in, 1 out]
            n130 = call "Subsystem_Name_To_File_Path_Or_NT_Variable.vi"("Enum String Name"="Climb") -> ("Names"=w235:string, "Values"=w234:string)  [unwired: 5 in, 1 out]
            n131 = call "Subsystem_Name_To_File_Path_Or_NT_Variable.vi"("Enum String Name"="Intake") -> ("Names"=w230:string, "Values"=w229:string)  [unwired: 5 in, 1 out]
            n132 = call "Subsystem_Name_To_File_Path_Or_NT_Variable.vi"("Enum String Name"="Flywheel") -> ("Names"=w225:string, "Values"=w224:string)  [unwired: 5 in, 1 out]
            n133 = call "Subsystem_Name_To_File_Path_Or_NT_Variable.vi"("Enum String Name"="Control_Panel_") -> ("Names"=w215:string, "Values"=w214:string)  [unwired: 5 in, 1 out]
            n134 = call-poly <vilib>:"NT Read Value.vi"("Name"=w245) -> ("String Array"=w243:string[])  [unwired: 9 in, 1 out]
            n135 = call-poly <vilib>:"NT Read Value.vi"("Name"=w244) -> ("String Array"=w242:string[])  [unwired: 9 in, 1 out]
            n136 = call-poly <vilib>:"NT Read Value.vi"("Name"=w220) -> ("String Array"=w218:string[])  [unwired: 9 in, 1 out]
            n137 = call-poly <vilib>:"NT Read Value.vi"("Name"=w219) -> ("String Array"=w217:string[])  [unwired: 9 in, 1 out]
            n138 = call-poly <vilib>:"NT Read Value.vi"("Name"=w240) -> ("String Array"=w238:string[])  [unwired: 9 in, 1 out]
            n139 = call-poly <vilib>:"NT Read Value.vi"("Name"=w239) -> ("String Array"=w237:string[])  [unwired: 9 in, 1 out]
            n140 = call-poly <vilib>:"NT Read Value.vi"("Name"=w235) -> ("String Array"=w233:string[])  [unwired: 9 in, 1 out]
            n141 = call-poly <vilib>:"NT Read Value.vi"("Name"=w230) -> ("String Array"=w228:string[])  [unwired: 9 in, 1 out]
            n142 = call-poly <vilib>:"NT Read Value.vi"("Name"=w234) -> ("String Array"=w232:string[])  [unwired: 9 in, 1 out]
            n143 = call-poly <vilib>:"NT Read Value.vi"("Name"=w229) -> ("String Array"=w227:string[])  [unwired: 9 in, 1 out]
            n144 = call-poly <vilib>:"NT Read Value.vi"("Name"=w225) -> ("String Array"=w223:string[])  [unwired: 9 in, 1 out]
            n145 = call-poly <vilib>:"NT Read Value.vi"("Name"=w215) -> ("String Array"=w213:string[])  [unwired: 9 in, 1 out]
            n146 = call-poly <vilib>:"NT Read Value.vi"("Name"=w224) -> ("String Array"=w222:string[])  [unwired: 9 in, 1 out]
            n147 = call-poly <vilib>:"NT Read Value.vi"("Name"=w214) -> ("String Array"=w212:string[])  [unwired: 9 in, 1 out]
            n148 = call "Read_From_NT_Into_Dashboard.vi"("Values Array"=w242, "Names Array"=w243, "Pages"=w247) -> ()  [unwired: 1 in]
            n149 = call "Read_From_NT_Into_Dashboard.vi"("Values Array"=w217, "Names Array"=w218, "Pages"=w207) -> ()  [unwired: 1 in]
            n150 = call "Read_From_NT_Into_Dashboard.vi"("Values Array"=w237, "Names Array"=w238, "Pages"=w211) -> ()  [unwired: 1 in]
            n151 = call "Read_From_NT_Into_Dashboard.vi"("Values Array"=w232, "Names Array"=w233, "Pages"=w210) -> ()  [unwired: 1 in]
            n152 = call "Read_From_NT_Into_Dashboard.vi"("Values Array"=w227, "Names Array"=w228, "Pages"=w209) -> ()  [unwired: 1 in]
            n153 = call "Read_From_NT_Into_Dashboard.vi"("Values Array"=w222, "Names Array"=w223, "Pages"=w208) -> ()  [unwired: 1 in]
            n154 = call "Read_From_NT_Into_Dashboard.vi"("Values Array"=w212, "Names Array"=w213, "Pages"=w206) -> ()  [unwired: 1 in]
            n155 = call-poly <vilib>:"NT Read Value.vi"("Name"="DriveCals") -> ()  [unwired: 9 in, 2 out]
            n156 = call-poly <vilib>:"NT Read Value.vi"("Name"="TurretCals") -> ()  [unwired: 9 in, 2 out]
            n157 = call-poly <vilib>:"NT Read Value.vi"("Name"="ClimbCals") -> ()  [unwired: 9 in, 2 out]
            n158 = call-poly <vilib>:"NT Read Value.vi"("Name"="IntakeCals") -> ()  [unwired: 9 in, 2 out]
            n159 = call-poly <vilib>:"NT Read Value.vi"("Name"="FlywheelCals") -> ()  [unwired: 9 in, 2 out]
            n160 = disable-structure shown="Disabled" {
              frame Disabled {
                n161 = Index Array() -> (element #1=w253, element #2=w254)  [unwired: 3 in]
                n162 = Spreadsheet String To Array(delimiter (Tab)=",", format string="%s", spreadsheet string=w253, array type (2D Dbl)=dbl[] []) -> (array=w259:dbl[])
                n163 = Spreadsheet String To Array(delimiter (Tab)=",", format string="%f", spreadsheet string=w254, array type (2D Dbl)=dbl[] []) -> (array=w260:dbl[])
                n164 = Build Array(w259, w260) -> (→"appended array":dbl[][])
              }
              frame Enabled {
              }
            }
          }
          frame "Write" {
            (unwired) enum32{"Controls", "Indicators"}."Controls" ("Climb")
            # "WIP"
            # "to get this thingy, double click on nested\ntab controls (the sections on the front \npanel), should go to tab control in \nblock diagram, right click there, go to\ncreate -> property node -> pages"
            n165 = property on="Turret" class="TabCtl (strict)"() -> ("Pages"=w303:refnum<vi>[])  [unwired: 2 in, 2 out]
            n166 = property on="Climb" class="TabCtl (strict)"() -> ("Pages"=w304:refnum<vi>[])  [unwired: 2 in, 2 out]
            n167 = property on="Intake" class="TabCtl (strict)"() -> ("Pages"=w305:refnum<vi>[])  [unwired: 2 in, 2 out]
            n168 = property on="Flywheel" class="TabCtl (strict)"() -> ("Pages"=w302:refnum<vi>[])  [unwired: 2 in, 2 out]
            n169 = property on="Magazine" class="TabCtl (strict)"() -> ("Pages"=w300:refnum<vi>[])  [unwired: 2 in, 2 out]
            n170 = property on="Control_Panel" class="TabCtl (strict)"() -> ("Pages"=w299:refnum<vi>[])  [unwired: 2 in, 2 out]
            n171 = property on="Drive" class="TabCtl (strict)"() -> ("Pages"=w301:refnum<vi>[])  [unwired: 2 in, 2 out]
            n172 = call "Write_From_Dash_Values_To_NT_Ready_Arrays.vi"("Pages"=w301) -> ("Names"=w277:string[], "Values"=w276:string[])
            n173 = call "Write_From_Dash_Values_To_NT_Ready_Arrays.vi"("Pages"=w299) -> ("Names"=w265:string[], "Values"=w264:string[])
            n174 = call "Write_From_Dash_Values_To_NT_Ready_Arrays.vi"("Pages"=w300) -> ("Names"=w267:string[], "Values"=w266:string[])
            n175 = call "Write_From_Dash_Values_To_NT_Ready_Arrays.vi"("Pages"=w303) -> ("Names"=w275:string[], "Values"=w274:string[])
            n176 = call "Write_From_Dash_Values_To_NT_Ready_Arrays.vi"("Pages"=w304) -> ("Names"=w273:string[], "Values"=w272:string[])
            n177 = call "Write_From_Dash_Values_To_NT_Ready_Arrays.vi"("Pages"=w302) -> ("Names"=w269:string[], "Values"=w268:string[])
            n178 = call "Write_From_Dash_Values_To_NT_Ready_Arrays.vi"("Pages"=w305) -> ("Names"=w271:string[], "Values"=w270:string[])
            n179 = call "Subsystem_Name_To_File_Path_Or_NT_Variable.vi"("Enum String Name"="Drive") -> ("Names"=w297:string, "Values"=w296:string)  [unwired: 5 in, 1 out]
            n180 = call "Subsystem_Name_To_File_Path_Or_NT_Variable.vi"("Enum String Name"="Turret") -> ("Names"=w294:string, "Values"=w293:string)  [unwired: 5 in, 1 out]
            n181 = call "Subsystem_Name_To_File_Path_Or_NT_Variable.vi"("Enum String Name"="Climb") -> ("Names"=w291:string, "Values"=w290:string)  [unwired: 5 in, 1 out]
            n182 = call "Subsystem_Name_To_File_Path_Or_NT_Variable.vi"("Enum String Name"="Intake") -> ("Names"=w288:string, "Values"=w287:string)  [unwired: 5 in, 1 out]
            n183 = call "Subsystem_Name_To_File_Path_Or_NT_Variable.vi"("Enum String Name"="Control_Panel_") -> ("Names"=w279:string, "Values"=w278:string)  [unwired: 5 in, 1 out]
            n184 = call "Subsystem_Name_To_File_Path_Or_NT_Variable.vi"("Enum String Name"="Flywheel") -> ("Names"=w285:string, "Values"=w284:string)  [unwired: 5 in, 1 out]
            n185 = call "Subsystem_Name_To_File_Path_Or_NT_Variable.vi"("Enum String Name"="Magazine") -> ("Names"=w282:string, "Values"=w281:string)  [unwired: 5 in, 1 out]
            n186 = call-poly <vilib>:"NT Write Value.vi"("String Array"=w277, "Name"=w297) -> ()  [unwired: 9 in, 1 out]
            n187 = call-poly <vilib>:"NT Write Value.vi"("String Array"=w276, "Name"=w296) -> ()  [unwired: 9 in, 1 out]
            n188 = call-poly <vilib>:"NT Write Value.vi"("String Array"=w275, "Name"=w294) -> ()  [unwired: 9 in, 1 out]
            n189 = call-poly <vilib>:"NT Write Value.vi"("String Array"=w274, "Name"=w293) -> ()  [unwired: 9 in, 1 out]
            n190 = call-poly <vilib>:"NT Write Value.vi"("String Array"=w273, "Name"=w291) -> ()  [unwired: 9 in, 1 out]
            n191 = call-poly <vilib>:"NT Write Value.vi"("String Array"=w272, "Name"=w290) -> ()  [unwired: 9 in, 1 out]
            n192 = call-poly <vilib>:"NT Write Value.vi"("String Array"=w271, "Name"=w288) -> ()  [unwired: 9 in, 1 out]
            n193 = call-poly <vilib>:"NT Write Value.vi"("String Array"=w270, "Name"=w287) -> ()  [unwired: 9 in, 1 out]
            n194 = call-poly <vilib>:"NT Write Value.vi"("String Array"=w265, "Name"=w279) -> ()  [unwired: 9 in, 1 out]
            n195 = call-poly <vilib>:"NT Write Value.vi"("String Array"=w264, "Name"=w278) -> ()  [unwired: 9 in, 1 out]
            n196 = call-poly <vilib>:"NT Write Value.vi"("String Array"=w269, "Name"=w285) -> ()  [unwired: 9 in, 1 out]
            n197 = call-poly <vilib>:"NT Write Value.vi"("String Array"=w268, "Name"=w284) -> ()  [unwired: 9 in, 1 out]
            n198 = call-poly <vilib>:"NT Write Value.vi"("String Array"=w267, "Name"=w282) -> ()  [unwired: 9 in, 1 out]
            n199 = call-poly <vilib>:"NT Write Value.vi"("String Array"=w266, "Name"=w281) -> ()  [unwired: 9 in, 1 out]
          }
        }
        n200 = call-poly <vilib>:"NT Read Value.vi"("Name"="Top_Middle_IR_Safety") -> ()  [unwired: 9 in, 2 out]
        "Drive" <- w181
        "Turret" <- w181
        "Climb" <- w181
        "Flywheel" <- w181
        "Intake" <- w181
        "Magazine" <- w181
        "Control_Panel" <- w181
      }
    }
  }
  n201 = register-events(refnum<vi> refnum, w25) -> (reference out=w62:refnum<event-registration>, error out=w61:errorcluster)  [unwired: 2 in]
  n202 = call "Initialize Camera and CheckList.vi"("ListBox in"=w46) -> ()  [unwired: 11 in]
  n203 = disable-structure shown="Disabled" {
    disable-tunnel: w57 -> [w309 _]
    disable-tunnel: w49 -> [w308 _]
    disable-tunnel: w47 -> [w307 _]
    disable-tunnel: w33 -> [w306 _]
    frame Disabled {
      n204 = call "Adjust Dashboard Window.vi"("Sizing Refnums"=w307, "Size Constraints"=w308, "VI"=w309, "WIn Mode"=w306) -> ()  [unwired: 8 in]
    }
    frame Enabled {
    }
  }
  n205 = vi-ref "Playback Controls.vi"() -> (w63:refnum<vi>)
  n206 = property class="VI"() -> ("Panel"=w65:refnum<vi>)  [unwired: 2 in, 2 out]
  n207 = while {
    tunnel: w73 -> [w323]
    tunnel: w72 -> [_]
    tunnel: w3 -> [w316]
    tunnel: w1 -> [w313]
    stop <- FALSE stop-if-true
    # "Optionally read the DB image,\nlog, or retrieve images from a\nlogged match"
    n208 = local read "NT Connection"() -> (w317:bool)
    n209 = local read "Rec Mode"() -> (w320:enum32{"Stop", "Record", "Playback"})
    n210 = local read "Right Camera Perf"() -> (w311:cluster{"Bandwidth (Mbps)":dbl, "FPS":dbl})
    n211 = Bundle("Camera Name"="Camera Name", w313, "Saved DB Images Info"=w316) -> (w315:T21)  [unwired: 1 in]
    n212 = control-ref of="Camera Perf"() -> (w310:refnum<vi>)
    n213 = call <vilib>:"WPI_CameraRead MJPG for Dashboard_2.vi"("Camera Settings"="Camera Settings", "Rec Mode"=w320, "NT Connection"=w317, "Capture Info"=w315, "Image in"=w323) -> ("perf info"=w312:cluster{"Bandwidth (Mbps)":dbl, "fps":dbl}, "Active"=w321:bool, "Image\\ out"=w322:T4)  [unwired: 4 in]
    n214 = case shown="True" w321 {
      tunnel: w322 -> [w326 w329]
      tunnel: [w326 w328] -> w318
      frame False {
        # "Sleep for 500ms"
        n215 = property on="Camera Image" class="ImageControl"("ROI"=T20 {"Global Rectangle"=[], "Contours"=[]}) -> ()  [unwired: 2 in, 2 out]
        n216 = Wait Until Next ms Multiple(millisecond multiple=u32 500) -> ()  [unwired: 1 out]
      }
      frame True {
        # "Here is where you would annotate,\npossibly process, and display the image"
        # "Update Mbps LED"
        n217 = call "IMAQ Clear Overlay"("Image"=w329) -> ("error out"=w330:errorcluster, "Image Out"=w328:T4)  [unwired: 2 in, 7 out]
        n218 = Unbundle By Name(w330) -> ("status"=w331:bool)
        n219 = property on="Image Message" class="Str"("Visible"=w331) -> ()  [unwired: 2 in, 2 out]
      }
    }
    "Camera Image" <- w318
    n220 = call <vilib>:"WPI_DashboardFormatPerf.vi"("Right Camera Perf"=w311, "Performance"=w312, "String in"=w310) -> ()  [unwired: 9 in]
  }
  n221 = while {
    tunnel: w12 -> [w346]
    tunnel: w11 -> [_]
    tunnel: [w341] -> _
    tunnel: w3 -> [w337]
    tunnel: w2 -> [w334]
    i -> [w341]
    stop <- FALSE stop-if-true
    n222 = local read "NT Connection"() -> (w338:bool)
    n223 = local read "Rec Mode"() -> (w345:enum32{"Stop", "Record", "Playback"})
    n224 = Bundle("Camera Name Right"="Camera Name Right", w334, "Saved DB Images Info"=w337) -> (w336:T22)  [unwired: 1 in]
    n225 = call <vilib>:"WPI_CameraRead MJPG for Dashboard_2.vi"("Camera Settings"="Camera Settings Right", "Rec Mode"=w345, "NT Connection"=w338, "Capture Info"=w336, "Image in"=w346) -> ("perf info"=w332:cluster{"Bandwidth (Mbps)":dbl, "fps":dbl}, "Active"=w340:bool, "Image\\ out"=w343:T4)  [unwired: 4 in]
    n226 = case shown="False" w340 {
      tunnel: w343 -> [w348 w351]
      tunnel: [w348 w351] -> w339
      tunnel: [_ w350] -> w333
      tunnel: w332 -> [_ w350]
      frame False {
        n227 = Wait Until Next ms Multiple(millisecond multiple=u32 500) -> ()  [unwired: 1 out]
        n228 = property on="Camera Image Right" class="ImageControl"("ROI"=T20 {"Global Rectangle"=[], "Contours"=[]}) -> ()  [unwired: 2 in, 2 out]
      }
      frame True {
      }
    }
    "Camera Image Right" <- w339
    "Right Camera Perf" <- w333
  }
  n229 = while {
    tunnel: w54 -> [w363]
    tunnel: w34 -> [w361]
    tunnel: [w359] -> _
    tunnel: u32 1000 ("milliseconds to wait") -> [w358]
    tunnel: w25 -> [w352]
    i -> [w359]
    stop <- FALSE stop-if-true
    n230 = local read "Rec Mode"() -> (w354:enum32{"Stop", "Record", "Playback"})
    n231 = Wait on Notification(notifier=w361, timeout in ms (-1)=w358) -> (notification=w360:string, timed out?=w356:bool)  [unwired: 2 in, 2 out]
    n232 = Equal?(x=w354, y=u16 2 ("Rec Mode")) -> (x = y?=w355:bool)
    n233 = Compound Arithmetic op=OR(invert w356, w355) -> (w357:bool)
    n234 = case shown="True" w357 {
      tunnel: w363 -> [_ w366]
      tunnel: w360 -> [_ w365]
      tunnel: w352 -> [_ w364]
      frame False {
      }
      frame True {
        n235 = call <vilib>:"Bind Controls to SmartDashboard.vi"("RPC ref"=w364, "Bound Control Refs"=w366, "Server IP Address"=w365) -> ()  [unwired: 9 in]
      }
    }
  }
  n236 = property class="Pnl"(reference=w65) -> ("Panes[]"=w66:refnum<vi>[])  [unwired: 1 in, 2 out]
  n237 = Index Array(array=w66) -> (element=w64:refnum<vi>)  [unwired: 1 in]
  n238 = control-ref of="Test Tree"() -> (w67:refnum<vi>)
  n239 = while {
    tunnel: [w376] -> _
    tunnel: w67 -> [w375]
    tunnel: w63 -> [w374]
    tunnel: w62 -> [w373]
    tunnel: w61 -> [_]
    tunnel: w57 -> [w372]
    tunnel: w25 -> [w371]
    tunnel: w23 -> [w370]
    shift-right: [w369] -> _
    shift-left: _ -> [w368]
    tunnel: w17 -> [w367]
    i -> [w376]
    stop <- FALSE stop-if-true
    n240 = event shown="[0] Timeout" {
      selector: w373 -> [_ _ _ _ _ _ _ _ _ _ _ _ _ _ _ _ _ _ _ _ _]
      dyn-events: [_ _ _ _ _ _ _ _ _ _ _ _ _ _ _ _ w636 _ _ _ _] -> _
      timeout: u32 60 ("milliseconds to wait") -> [_ _ _ _ _ _ _ _ _ _ _ _ _ _ _ _ _ _ _ _ _]
      tunnel: w375 -> [w388 _ _ _ _ _ _ _ _ _ _ _ _ _ _ _ _ _ _ _ _]
      tunnel: "Test Tree" -> [_ _ _ _ _ _ _ _ _ _ _ w603 w611 w613 w617 w625 _ _ _ _ _]
      tunnel: w374 -> [_ _ _ _ _ _ _ _ _ _ _ _ _ _ _ _ w638 _ w656 _ _]
      tunnel: w372 -> [_ _ _ _ _ _ _ _ _ _ _ _ _ _ _ _ w634 _ _ _ _]
      tunnel: w371 -> [_ _ _ _ _ _ _ _ _ _ _ _ _ _ _ _ w632 _ _ _ _]
      tunnel: w370 -> [w383 _ _ _ _ _ w554 _ _ _ _ _ _ _ _ _ _ _ _ _ _]
      tunnel: [w382 w431 w533 w538 w547 w551 w552 w561 w571 w578 w590 w602 w609 w612 w616 w624 w631 w651 w653 w657 w670] -> w369
      tunnel: w368 -> [w382 w431 w533 w538 w547 w551 w552 _ _ w578 w590 w602 w609 w612 w616 w624 w631 w651 w653 w657 w670]
      tunnel: w367 -> [w380 _ _ _ _ _ _ _ _ _ _ _ _ _ _ _ _ _ _ _ _]
      event Timeout {
        n241 = event-data() -> ()  [unwired: 1 in, 1 out]
        n242 = local read "Mode"() -> (w385:T3)
        n243 = case shown="\"Basic\"" "Dashboard Tab" {
          tunnel: w388 -> [_ _ w404 _ _]
          tunnel: "TestMode/Automatic/" ("Name Pattern") -> [_ _ w403 _ _]
          tunnel: T23 [{"Operation"=enum."Clear", "Color Box"=14013909}, {"Operation"=enum."Clear", "Color Box"=14013909}, {"Operation"=enum."Clear", "Color Box"=14013909}, {"Operation"=enum."Clear", "Color Box"=14013909}, {"Operation"=enum."Update", "Color Box"=14013909}, {"Operation"=enum."Update", "Color Box"=16777215}, {"Operation"=enum."Clear", "Color Box"=14013909}, {"Operation"=enum."Clear", "Color Box"=14013909}, {"Operation"=enum."Clear", "Color Box"=14013909}] -> [_ _ w396 _ w424]
          tunnel: w385 -> [_ _ w395 _ w423]
          tunnel: u32[] [15790320, 15790320, 15790320, 15790320, 16777215, 16777215, 15790320, 15790320, 15790320] -> [_ _ _ _ w429]
          tunnel: w383 -> [_ _ _ _ w417]
          tunnel: w380 -> [_ w390 _ _ _]
          frame "Custom", Default {
          }
          frame "Basic" {
            n244 = call <vilib>:"WPI_DashboardUpdateNames.vi"("Controls on Tab"=w390) -> ()  [unwired: 11 in]
          }
          frame "Test" {
            w402 = -2 ("Active Item:Row Number")
            n245 = Index Array(array=w396, index=w395) -> (element=w397:T26)
            n246 = Unbundle(w397) -> ("Operation"=w398:enum16{"Update", "Clear"}, "Color Box"=w399:u32)
            n247 = call <vilib>:"NT Read String.vi"("Name"="TestMode/TestName") -> ("String"=w393:string)  [unwired: 9 in, 1 out]
            n248 = call <vilib>:"NT Read and Format Entries as Tree.vi"("Operation"=w398, "Name Pattern"=w403, "Tree Refnum"=w404) -> ()  [unwired: 7 in, 2 out]
            n249 = case shown="\"\"" w393 {
              tunnel: "TestMode/TestProgress" ("Name") -> [w406 _]
              tunnel: "TestMode/TestProgressText" ("Name") -> [w405 _]
              frame Default {
                n250 = call <vilib>:"NT Read Number.vi"("Name"=w406) -> ("Numeric"=w407:dbl)  [unwired: 9 in, 1 out]
                n251 = call <vilib>:"NT Read String.vi"("Name"=w405) -> ("String"=w408:string)  [unwired: 9 in, 1 out]
                n252 = Bundle("Numeric"=w407, "String"=w408) -> (→"Progress":cluster{"Numeric":dbl, "String":string})  [unwired: 1 in]
              }
              frame "" {
                n253 = property on="Progress" class="Clust (strict)"("Visible"=FALSE) -> ()  [unwired: 2 in, 2 out]
                n254 = local write "Test Name"(u16 0) -> ()
              }
            }
            n255 = property on="Test Tree" class="Tree (strict)"("Active Item Row Number"=w402, "ActiveColNum"=w402, "CellBG"=w399, "Active Item Row Number"=-1 ("Active Item:Row Number"), "CellBG"=u32 5789784 ("Color Box")) -> ()  [unwired: 2 in, 2 out]
          }
          frame "Variables" {
            w414 = string[] ["CameraPublisher", "Usage", "DB"]  # Items to initially close
            n256 = First Call?() -> (First Call?: T/F=w415:bool)
            n257 = control-ref of="Tree"() -> (w416:refnum<vi>)
            n258 = Select(t=w414, s=w415, f=string[] []) -> (s? t:f=w412:string[])
            n259 = call <vilib>:"NT Read and Format Entries as Tree.vi"("Tags to  Close"=w412, "Tree Refnum"=w416) -> ()  [unwired: 8 in, 2 out]
          }
          frame "Commands" {
            w425 = u32 5789784 ("Color Box")
            w426 = T27 {"Row"=-1, "Column"=-2} ("Active Cell:Active Cell")
            w428 = T27 {"Row"=-2, "Column"=-2} ("Active Cell:Active Cell")
            n260 = Index Array(array=w429, index=w423) -> (element=w427:u32)
            n261 = Index Array(array=w424, index=w423) -> (element=w422:T26)
            n262 = Unbundle(w422) -> ("Operation"=w421:enum16{"Update", "Clear"})  [unwired: 1 out]
            n263 = local read "Command Selection"() -> (w420:i32)
            n264 = property on="Command Selection" class="MCListbox (strict)"("ActiveCell"=w428, "CellBG"=w427, "ActiveCell"=w426, "CellBG"=w425) -> ()  [unwired: 2 in, 2 out]
            n265 = call <vilib>:"WPI_DashboardUpdate RPC Info.vi"("Operation"=w421) -> ("update"=w419:bool, "commands"=w418:string[][])  [unwired: 9 in]
            n266 = property on="Command Selection" class="MCListbox (strict)"("ItemNames"=w418) -> ()  [unwired: 2 in, 2 out]
            n267 = property on="Command Params" class="Tbl (strict)"("Active Cell"=w428, "Cell BG Color"=w427, "Active Cell"=w426, "Cell BG Color"=w425) -> ()  [unwired: 2 in, 2 out]
            n268 = call <vilib>:"WPI_DashboardUpdate Command Params.vi"("Update"=w419, "NewVal"=w420, "Commands"=w418, "Param Tbl"=w417) -> ()  [unwired: 7 in, 1 out]
          }
        }
        n269 = call <vilib>:"Connextion Info.vi"() -> ("Connected"=→"NT Connection":bool)  [unwired: 10 in, 1 out]
      }
      event "Test Tree": Value Change {
        # "Show appropriate\ncontrols"
        n270 = event-data() -> ("CtlRef"=w434:refnum<vi>, "NewVal"=w432:string)  [unwired: 1 in]
        n271 = call <vilib>:"WPI_UtilitiesGetTreeIOName.vi"("NewVal"=w432, "TreeControl in"=w434) -> ("I/O Name"=w435:string)  [unwired: 9 in]
        n272 = case shown="\"Camera\"" w435 {
          selector: w435 -> [_ w442 _ w464 w473 _]
          tunnel: w432 -> [_ _ w461 w463 _ w480]
          tunnel: cluster{string[]}[] [{["640x480", "320x240", "160x120"]}, {["Auto", "Fixed indoor", "Fixed outdoor 1", "Fixed outdoor 2", "Fixed fluorescent 1", "Fixed fluorescent 2", "Hold current"]}, {["Auto", "Flicker-free 50 Hz", "Flicker-free 60 Hz", "Hold current"]}, {["None", "Prioritize frame rate", "Prioritize image quality"]}, {["Monochrome", "Color"]}] -> [_ _ _ _ _ w479]
          frame Default {
            w437 = FALSE ("Visible")
            w436 = FALSE ("Visible")
            n273 = property on="Motor" class="Clust (strict)"("Visible"=w436) -> ()  [unwired: 2 in, 2 out]
            n274 = property on="Test Ring" class="Ring (strict)"("Visible"=w436) -> ()  [unwired: 2 in, 2 out]
            n275 = property on="Rev/Fwd" class="Clust (strict)"("Visible"=w437) -> ()  [unwired: 2 in, 2 out]
            n276 = property on="On/Off" class="Bool (strict)"("Visible"=w437) -> ()  [unwired: 2 in, 2 out]
            n277 = property on="Test Slider" class="Slide (strict)"("Visible"=w437) -> ()  [unwired: 2 in, 2 out]
          }
          frame "Analog Out", "Motor", "PWM" {
            w443 = FALSE ("Visible")
            n278 = case shown="\"Analog Out\"" w442 {
              tunnel: [1.0 ("Value") -1.0 ("Value") 0.0 ("Value")] -> w441
              tunnel: [255.0 ("Value") 1.0 ("Value") 5.0 ("Value")] -> w440
              tunnel: [128.0 ("Value") 0.0 ("Value") 0.0 ("Value")] -> w439
              tunnel: [64.0 ("Value") 0.5 ("Value") 1.0 ("Value")] -> w438
              frame "PWM" {
              }
              frame "Motor", Default {
              }
              frame "Analog Out" {
              }
            }
            n279 = property on="Motor" class="Clust (strict)"("Visible"=TRUE) -> ()  [unwired: 2 in, 2 out]
            n280 = property on="Value" class="Slide (strict)"("Value"=w439, "Scale.Minimum"=w441, "Scale.Maximum"=w440, "Scale.Increment"=w438) -> ()  [unwired: 2 in, 2 out]
            n281 = property on="On/Off" class="Bool (strict)"("Visible"=w443) -> ()  [unwired: 2 in, 2 out]
            n282 = property on="Test Slider" class="Slide (strict)"("Visible"=w443) -> ()  [unwired: 2 in, 2 out]
            n283 = property on="Test Ring" class="Ring (strict)"("Visible"=w443) -> ()  [unwired: 2 in, 2 out]
            n284 = property on="Rev/Fwd" class="Clust (strict)"("Visible"=w443) -> ()  [unwired: 2 in, 2 out]
          }
          frame "Servo" {
            w459 = FALSE ("Visible")
            n285 = call <vilib>:"NT Read Number.vi"("Name"=w461) -> ("Numeric"=w460:dbl)  [unwired: 9 in, 1 out]
            n286 = property on="Test Slider" class="Slide (strict)"("Visible"=TRUE, "Scale.Maximum"=170.0 ("Scale.Range:Maximum")) -> ()  [unwired: 2 in, 2 out]
            n287 = local write "Test Slider"(w460) -> ()
            n288 = property on="Motor" class="Clust (strict)"("Visible"=w459) -> ()  [unwired: 2 in, 2 out]
            n289 = property on="Rev/Fwd" class="Clust (strict)"("Visible"=w459) -> ()  [unwired: 2 in, 2 out]
            n290 = property on="On/Off" class="Bool (strict)"("Visible"=w459) -> ()  [unwired: 2 in, 2 out]
            n291 = property on="Test Ring" class="Ring (strict)"("Visible"=w459) -> ()  [unwired: 2 in, 2 out]
          }
          frame "Relay", "Solenoid" {
            w462 = FALSE ("Visible")
            n292 = property on="Motor" class="Clust (strict)"("Visible"=w462) -> ()  [unwired: 2 in, 2 out]
            n293 = property on="Test Slider" class="Slide (strict)"("Visible"=w462) -> ()  [unwired: 2 in, 2 out]
            n294 = Search and Replace String(input string=w463, search string="/Value  **", replace string="/Direction") -> (result string=w469:string)  [unwired: 5 in, 3 out]
            n295 = property on="Test Ring" class="Ring (strict)"("Visible"=w462) -> ()  [unwired: 2 in, 2 out]
            n296 = call <vilib>:"NT Read String.vi"("Name"=w469) -> ("String"=w467:string)  [unwired: 9 in, 1 out]
            n297 = Equal?(x="Both directions", y=w467) -> (x = y?=w465:bool)
            n298 = Not(x=w465) -> (.not. x?=w466:bool)
            n299 = property on="Rev/Fwd" class="Clust (strict)"("Visible"=w465) -> ()  [unwired: 2 in, 2 out]
            n300 = property on="On/Off" class="Bool (strict)"("Visible"=w466, "Caption.Text"=w464) -> ()  [unwired: 2 in, 2 out]
          }
          frame "Compressor", "Digital Out" {
            w472 = FALSE ("Visible")
            # "Get direction and finish"
            n301 = property on="Motor" class="Clust (strict)"("Visible"=w472) -> ()  [unwired: 2 in, 2 out]
            n302 = property on="Test Slider" class="Slide (strict)"("Visible"=w472) -> ()  [unwired: 2 in, 2 out]
            n303 = property on="Test Ring" class="Ring (strict)"("Visible"=w472) -> ()  [unwired: 2 in, 2 out]
            n304 = property on="On/Off" class="Bool (strict)"("Visible"=TRUE, "Caption.Text"=w473) -> ()  [unwired: 2 in, 2 out]
            n305 = property on="Rev/Fwd" class="Clust (strict)"("Visible"=FALSE) -> ()  [unwired: 2 in, 2 out]
          }
          frame "Camera" {
            n306 = call <vilib>:"Get Last Path Segment.vi"("String in"=w480) -> ("String out"=w481:string)  [unwired: 10 in]
            n307 = property on="On/Off" class="Bool (strict)"("Visible"=FALSE) -> ()  [unwired: 2 in, 2 out]
            n308 = property on="Motor" class="Clust (strict)"("Visible"=FALSE) -> ()  [unwired: 2 in, 2 out]
            n309 = property on="Rev/Fwd" class="Clust (strict)"("Visible"=FALSE) -> ()  [unwired: 2 in, 2 out]
            n310 = case shown="\"White Balance  **\"" w481 {
              tunnel: w480 -> [w487 w496 w505 w514 w523 _ w529]
              tunnel: w479 -> [w485 w493 w502 w511 w520 _ _]
              frame "Size  **" {
                n311 = Index Array(array=w485) -> (element=w484:cluster{string[]})  [unwired: 1 in]
                n312 = call <vilib>:"NT Read String.vi"("Name"=w487) -> ("String"=w486:string)  [unwired: 9 in, 1 out]
                n313 = Unbundle(w484) -> (w482:string[])
                n314 = Match First String(2:w482, 3:w486) -> (0:w483:i32)  [unwired: 1 out]
                n315 = property on="Test Ring" class="Ring (strict)"("Value"=w483, "Strings []"=w482) -> ()  [unwired: 2 in, 2 out]
                n316 = property on="Test Ring" class="Ring (strict)"("Visible"=TRUE) -> ()  [unwired: 2 in, 2 out]
                n317 = property on="Test Slider" class="Slide (strict)"("Visible"=FALSE) -> ()  [unwired: 2 in, 2 out]
              }
              frame "White Balance  **" {
                n318 = Index Array(array=w493, index=1) -> (element=w494:cluster{string[]})
                n319 = call <vilib>:"NT Read String.vi"("Name"=w496) -> ("String"=w495:string)  [unwired: 9 in, 1 out]
                n320 = Unbundle(w494) -> (w491:string[])
                n321 = Match First String(2:w491, 3:w495) -> (0:w490:i32)  [unwired: 1 out]
                n322 = property on="Test Ring" class="Ring (strict)"("Value"=w490, "Strings []"=w491) -> ()  [unwired: 2 in, 2 out]
                n323 = property on="Test Ring" class="Ring (strict)"("Visible"=TRUE) -> ()  [unwired: 2 in, 2 out]
                n324 = property on="Test Slider" class="Slide (strict)"("Visible"=FALSE) -> ()  [unwired: 2 in, 2 out]
              }
              frame "Exposure  **" {
                n325 = Index Array(array=w502, index=2) -> (element=w503:cluster{string[]})
                n326 = call <vilib>:"NT Read String.vi"("Name"=w505) -> ("String"=w504:string)  [unwired: 9 in, 1 out]
                n327 = Unbundle(w503) -> (w499:string[])
                n328 = Match First String(2:w499, 3:w504) -> (0:w500:i32)  [unwired: 1 out]
                n329 = property on="Test Ring" class="Ring (strict)"("Value"=w500, "Strings []"=w499) -> ()  [unwired: 2 in, 2 out]
                n330 = property on="Test Ring" class="Ring (strict)"("Visible"=TRUE) -> ()  [unwired: 2 in, 2 out]
                n331 = property on="Test Slider" class="Slide (strict)"("Visible"=FALSE) -> ()  [unwired: 2 in, 2 out]
              }
              frame "Exposure Priority  **" {
                n332 = Index Array(array=w511, index=3) -> (element=w512:cluster{string[]})
                n333 = call <vilib>:"NT Read String.vi"("Name"=w514) -> ("String"=w513:string)  [unwired: 9 in, 1 out]
                n334 = Unbundle(w512) -> (w508:string[])
                n335 = Match First String(2:w508, 3:w513) -> (0:w509:i32)  [unwired: 1 out]
                n336 = property on="Test Ring" class="Ring (strict)"("Value"=w509, "Strings []"=w508) -> ()  [unwired: 2 in, 2 out]
                n337 = property on="Test Ring" class="Ring (strict)"("Visible"=TRUE) -> ()  [unwired: 2 in, 2 out]
                n338 = property on="Test Slider" class="Slide (strict)"("Visible"=FALSE) -> ()  [unwired: 2 in, 2 out]
              }
              frame "Color Enable  **" {
                n339 = Index Array(array=w520, index=4) -> (element=w521:cluster{string[]})
                n340 = call <vilib>:"NT Read String.vi"("Name"=w523) -> ("String"=w522:string)  [unwired: 9 in, 1 out]
                n341 = Unbundle(w521) -> (w517:string[])
                n342 = Match First String(2:w517, 3:w522) -> (0:w518:i32)  [unwired: 1 out]
                n343 = property on="Test Ring" class="Ring (strict)"("Value"=w518, "Strings []"=w517) -> ()  [unwired: 2 in, 2 out]
                n344 = property on="Test Ring" class="Ring (strict)"("Visible"=TRUE) -> ()  [unwired: 2 in, 2 out]
                n345 = property on="Test Slider" class="Slide (strict)"("Visible"=FALSE) -> ()  [unwired: 2 in, 2 out]
              }
              frame Default {
                n346 = property on="Test Ring" class="Ring (strict)"("Visible"=FALSE) -> ()  [unwired: 2 in, 2 out]
                n347 = property on="Test Slider" class="Slide (strict)"("Visible"=FALSE) -> ()  [unwired: 2 in, 2 out]
              }
              frame "Brightness  **", "Color Level  **", "Compression  **", "FPS  **", "Sharpness  **" {
                n348 = call <vilib>:"NT Read Number.vi"("Name"=w529) -> ("Numeric"=w528:dbl)  [unwired: 9 in, 1 out]
                n349 = local write "Test Slider"(w528) -> ()
                n350 = property on="Test Slider" class="Slide (strict)"("Visible"=TRUE, "Scale.Maximum"=100.0 ("Scale.Range:Maximum")) -> ()  [unwired: 2 in, 2 out]
                n351 = property on="Test Ring" class="Ring (strict)"("Visible"=FALSE) -> ()  [unwired: 2 in, 2 out]
              }
            }
          }
        }
        n352 = property on="Progress" class="Clust (strict)"("Visible"=FALSE) -> ()  [unwired: 2 in, 2 out]
      }
      event "Test Name": Mouse Enter {
        # "Populate the ring with the list of tests"
        n353 = event-data() -> ()  [unwired: 1 in, 1 out]
        n354 = call <vilib>:"NT Read String Array.vi"("Name"="TestMode/TestList") -> ("String Array"=w537:string[])  [unwired: 9 in, 1 out]
        n355 = Build Array (concatenate)("Select the test to run...", w537) -> (w536:string[])
        n356 = property on="Test Name" class="Ring (strict)"("Strings []"=w536) -> ()  [unwired: 2 in, 2 out]
      }
      event "Test Name": Value Change {
        w539 = FALSE ("Visible")
        # "Tell the robot the test name to run"
        n357 = event-data() -> ("NewVal"=w543:u16)  [unwired: 1 in]
        n358 = property on="Test Name" class="Ring (strict)"() -> ("Strings []"=w544:string[])  [unwired: 2 in, 2 out]
        n359 = local write "Progress"(T6 {"Test Progress"=0, "Test Progress Text"=""} ("Progress")) -> ()
        n360 = Index Array(array=w544, index=w543) -> (element=w542:string)
        n361 = call <vilib>:"NT Write String.vi"("String"=w542, "Name"="TestMode/TestName") -> ()  [unwired: 9 in, 1 out]
        n362 = property on="Progress" class="Clust (strict)"("Visible"=TRUE) -> ()  [unwired: 2 in, 2 out]
        n363 = property on="Motor" class="Clust (strict)"("Visible"=w539) -> ()  [unwired: 2 in, 2 out]
        n364 = property on="Test Slider" class="Slide (strict)"("Visible"=w539) -> ()  [unwired: 2 in, 2 out]
        n365 = property on="On/Off" class="Bool (strict)"("Visible"=w539) -> ()  [unwired: 2 in, 2 out]
        n366 = property on="Rev/Fwd" class="Clust (strict)"("Visible"=w539) -> ()  [unwired: 2 in, 2 out]
        n367 = property on="Test Ring" class="Ring (strict)"("Visible"=w539) -> ()  [unwired: 2 in, 2 out]
      }
      event "Select Auto": Mouse Enter {
        # "Populate the combo box with the list of autonomous options"
        n368 = event-data() -> ()  [unwired: 1 in, 1 out]
        n369 = call <vilib>:"NT Read String Array.vi"("Name"="Auto List") -> ("String Array"=w546:string[])  [unwired: 9 in, 1 out]
        n370 = property on="Select Auto" class="CmbBox"("Strings[]"=w546) -> ()  [unwired: 2 in, 2 out]
      }
      event "Select Auto": Value Change {
        # "User modified the Auto Selection. Write to NT variable so robot knows."
        n371 = event-data() -> ("NewVal"=w549:string)  [unwired: 1 in]
        n372 = call <vilib>:"NT Write String.vi"("String"=w549, "Name"="Auto Selector") -> ()  [unwired: 9 in, 1 out]
      }
      event "Command Selection": Value Change {
        # "Get the params and show in table"
        n373 = event-data() -> ("NewVal"=w555:i32)  [unwired: 1 in]
        n374 = property on="Command Selection" class="MCListbox (strict)"() -> ("ItemNames"=w553:string[][])  [unwired: 2 in, 2 out]
        n375 = call <vilib>:"WPI_DashboardUpdate Command Params.vi"("NewVal"=w555, "Commands"=w553, "Param Tbl"=w554) -> ()  [unwired: 8 in, 1 out]
      }
      event "Execute Command": Value Change {
        # "Started one, Unique ID holds\nresponse"
        n376 = event-data() -> ()  [unwired: 1 in, 1 out]
        n377 = property on="Command Selection" class="MCListbox (strict)"() -> ("ItemNames"=w566:string[][])  [unwired: 2 in, 2 out]
        n378 = Index Array(array=w566, index (row)="Command Selection", index (col)=0) -> (element=w564:string)
        n379 = call <vilib>:"Invoke Commands.vi"("Command Params"="Command Params", "Function Name"=w564) -> ("Params"=w560:u8, "Started"=w559:bool)  [unwired: 7 in, 1 out]
        n380 = Array Subset(array="Command Params", length (row)=w560) -> (w561:string[][])  [unwired: 3 in]
        n381 = Select(t="Executing" ("Cmd Status"), s=w559, f="" ("Cmd Status")) -> (s? t:f=→"Cmd Status":string)
      }
      event "Command Selection": Double Click {
        n382 = event-data() -> ("Row"=w574:i32)  [unwired: 1 in]
        n383 = property on="Command Selection" class="MCListbox (strict)"() -> ("ItemNames"=w577:string[][])  [unwired: 2 in, 2 out]
        n384 = local read "Command Params"() -> (w573:string[][])
        n385 = Index Array(array=w577, index (row)=w574, index (col)=0) -> (element=w575:string)
        n386 = call <vilib>:"Invoke Commands.vi"("Command Params"=w573, "Function Name"=w575) -> ("Params"=w572:u8, "Started"=w567:bool)  [unwired: 7 in, 1 out]
        n387 = Array Subset(array=w573, length (row)=w572) -> (w571:string[][])  [unwired: 3 in]
        n388 = Select(t="Executing" ("Cmd Status"), s=w567, f="" ("Cmd Status")) -> (s? t:f=w568:string)
        n389 = local write "Cmd Status"(w568) -> ()
      }
      event "CheckList": Double Click {
        # "Shift clears all"
        # "Update symbols on the listbox"
        n390 = event-data() -> ("PlatMods.Shift"=w579:bool, "Row"=w581:i32)  [unwired: 1 in]
        n391 = case shown="True" w579 {
          tunnel: w581 -> [w585 _]
          tunnel: 1 -> [w584 _]
          frame False {
            n392 = property on="CheckList" class="LstBox (strict)"() -> ("Item Symbols"=w583:i32[])  [unwired: 2 in, 2 out]
            n393 = Replace Array Subset(array=w583, new element=w584, index=w585) -> (w582:i32[])
            n394 = property on="CheckList" class="LstBox (strict)"("Item Symbols"=w582) -> ()  [unwired: 2 in, 2 out]
          }
          frame True {
            w586 = 0 ("Top Row")
            n395 = property on="CheckList" class="LstBox (strict)"() -> ("Number of Rows"=w588:u32)  [unwired: 2 in, 2 out]
            n396 = Initialize Array(0, w588) -> (w587:i32[])
            n397 = property on="CheckList" class="LstBox (strict)"("Top Row"=w586, "Value"=w586, "Item Symbols"=w587) -> ()  [unwired: 2 in, 2 out]
          }
        }
      }
      event "CheckList": Key Down {
        # "Update symbols on the listbox\nLeft and right keys check and uncheck"
        n398 = event-data() -> ("VKey"=w592:T24)  [unwired: 1 in]
        n399 = case shown="\"Left\", \"Right\"" w592 {
          selector: w592 -> [w597 _]
          tunnel: eventvkey."Left" ("VKey") -> [w595 _]
          frame "Left", "Right" {
            n400 = Equal?(x=w595, y=w597) -> (x = y?=w596:bool)
            n401 = Select(t=0, s=w596, f=1) -> (s? t:f=w598:i32)
            n402 = property on="CheckList" class="LstBox (strict)"() -> ("Item Symbols"=w601:i32[])  [unwired: 2 in, 2 out]
            n403 = Replace Array Subset(array=w601, new element=w598, index="CheckList") -> (w600:i32[])
            n404 = property on="CheckList" class="LstBox (strict)"("Item Symbols"=w600) -> ()  [unwired: 2 in, 2 out]
          }
          frame Default {
          }
        }
      }
      event "Motor.Enable": Value Change {
        # "When the test mode otor enable helper is set, update that\ntree row item's value"
        n405 = event-data() -> ("NewVal"=w607:bool)  [unwired: 1 in]
        n406 = Unbundle("Motor") -> ("Value"=w606:dbl)  [unwired: 1 out]
        n407 = Select(t=w606, s=w607, f=0.0) -> (s? t:f=w604:dbl)
        n408 = call <vilib>:"NT Write Number.vi"("Numeric"=w604, "Name"=w603) -> ()  [unwired: 9 in, 1 out]
      }
      event "Test Slider": Value Change {
        # "When the test mode slider helper is set, update that\ntree row item's value"
        n409 = event-data() -> ("NewVal"=w610:dbl)  [unwired: 1 in]
        n410 = call <vilib>:"NT Write Number.vi"("Numeric"=w610, "Name"=w611) -> ()  [unwired: 9 in, 1 out]
      }
      event "On/Off": Value Change {
        # "When the test mode on/off helper value is set, update that\ntree row item's value"
        n411 = event-data() -> ("NewVal"=w615:bool)  [unwired: 1 in]
        n412 = Boolean To (0,1)(Boolean=w615) -> (0, 1=w614:i16)
        n413 = call <vilib>:"NT Write Number.vi"("Numeric"=w614, "Name"=w613) -> ()  [unwired: 9 in, 1 out]
      }
      event "Rev/Fwd": Value Change {
        # "When the test mode helper value for relays is set, update that\ntree row item's value"
        n414 = event-data() -> ("NewVal.Forward"=w623:bool, "NewVal.Reverse"=w622:bool)  [unwired: 1 in]
        n415 = Boolean To (0,1)(Boolean=w623) -> (0, 1=w619:i16)
        n416 = Boolean To (0,1)(Boolean=w622) -> (0, 1=w621:i16)
        n417 = Negate(x=w621) -> (-x=w620:i16)
        n418 = Add(x=w619, y=w620) -> (x+y=w618:i16)
        n419 = call <vilib>:"NT Write Number.vi"("Numeric"=w618, "Name"=w617) -> ()  [unwired: 9 in, 1 out]
      }
      event "Test Ring": Value Change {
        # "When a test mode helper value is selected from the ring,\nset the tree item's variable to the string value"
        n420 = event-data() -> ("NewVal"=w627:u16)  [unwired: 1 in]
        n421 = property on="Test Ring" class="Ring (strict)"() -> ("Strings []"=w628:string[])  [unwired: 2 in, 2 out]
        n422 = Index Array(array=w628, index=w627) -> (element=w626:string)
        n423 = call <vilib>:"NT Write String.vi"("String"=w626, "Name"=w625) -> ()  [unwired: 9 in, 1 out]
      }
      event "Rec Mode": Value Change {
        # "Update globals for recording mode and path to read log from.\nClear when logging and let NetworkTables set path for vision to\nuse."
        n424 = event-data() -> ("NewVal"=w639:enum32{"Stop", "Record", "Playback"})  [unwired: 1 in]
        n425 = global write "WPI_DashboardLogging Global.vi" "Logging Filename"(path "") -> ()
        n426 = global write "WPI_DashboardLogging Global.vi" "Recording"(w639) -> ()
        n427 = case shown="\"Playback\"" w639 {
          tunnel: w638 -> [_ w641 w650]
          tunnel: [_ _ w649] -> w636
          tunnel: [_ _ w648] -> _
          tunnel: w634 -> [_ _ w646]
          tunnel: cluster{i32, i32} {-250, 170} -> [_ _ w645]
          tunnel: [_ _ T25 {"Image Size"=TRUE, "Image Type"=TRUE, "Pixel Value"=TRUE, "ROI Information"=TRUE, "Zoom Factor"=FALSE} ("Image Information Shown:All Elements")] -> w629
          tunnel: [_ _ TRUE ("Zoom Factor")] -> w630
          tunnel: w632 -> [_ _ w642]
          frame Default {
          }
          frame "Stop", "Record" {
            # "Place Window too"
            n428 = invoke class="VI" method="FP.Close"(reference=w641) -> (reference out=w640:refnum<vi>)  [unwired: 2 in, 2 out]
            n429 = invoke class="VI" method="Abort VI"(reference=w640) -> ()  [unwired: 2 in, 3 out]
          }
          frame "Playback" {
            n430 = call "Open Playback Panel.vi"("Offset"=w645, "DB VI Ref"=w646, "Playback in"=w650) -> ("Playback out"=w647:refnum<vi>)  [unwired: 8 in]
            n431 = register-events(w647, w642) -> (reference out=w649:refnum<event-registration>, error out=w648:errorcluster)  [unwired: 2 in]
          }
        }
        n432 = property on="Camera Image Right" class="ImageControl"("Image Information Shown"=w629, "Image Information Visible"=w630) -> ()  [unwired: 2 in, 2 out]
        n433 = property on="Camera Image" class="ImageControl"("Image Information Shown"=w629, "Image Information Visible"=w630) -> ()  [unwired: 2 in, 2 out]
        n434 = call <vilib>:"WPI_DashboardNT Log FieldName Cache.vi"("Operation"=enum16{"Lookup/Add", "Index", "Clear"}."Clear") -> ()  [unwired: 8 in, 3 out]
      }
      event Panel Close {
        w652 = enum32{"Stop", "Record", "Playback"}."Stop" ("Rec Mode")
        # "Playback window has been closed, abort"
        n435 = event-data() -> ()  [unwired: 1 in, 4 out]
        n436 = local write "Rec Mode"(w652) -> ()
        n437 = global write "WPI_DashboardLogging Global.vi" "Recording"(w652) -> ()
      }
      event Panel Close {
        # "Abort playback window and ourself"
        n438 = event-data() -> ()  [unwired: 1 in, 4 out]
        n439 = invoke class="VI" method="FP.Close"(reference=w656) -> (reference out=w655:refnum<vi>)  [unwired: 2 in, 2 out]
        n440 = invoke class="VI" method="Abort VI"(reference=w655) -> (error out=w654:errorcluster)  [unwired: 2 in, 2 out]
        n441 = invoke class="VI" method="Abort VI"(error in=w654) -> ()  [unwired: 2 in, 3 out]
      }
      event User Event {
        n442 = event-data() -> ("IDs"=w663:cluster{"RPC field ID":u16, "Unique ID":u16}, "String"=w662:string)  [unwired: 1 in]
        n443 = Bundle("IDs"=w663, "String"=w662) -> (w661:T11)  [unwired: 1 in]
        n444 = call <vilib>:"Retrieve RPC Response.vi"("RPC Response"=w661) -> ("Output"=w659:string[][])  [unwired: 10 in]
        n445 = Build Array (concatenate)(w657, w659) -> (w658:string[][])
        n446 = local write "Command Params"(w658) -> ()
        n447 = local write "Cmd Status"("" ("Cmd Status")) -> ()
      }
      event "Tree": Double Click {
        n448 = event-data() -> ("PlatMods"=w669:T28, "Tag"=w666:string)  [unwired: 1 in]
        n449 = Unbundle(w669) -> ("Shift"=w668:bool)  [unwired: 4 out]
        n450 = String Subset(string=w666, length (rest)=1 ("length (rest)")) -> (substring=w665:string)  [unwired: 1 in]
        n451 = Not(x=w668) -> (.not. x?=w667:bool)
        n452 = case shown="\"/\"" w665 {
          tunnel: w666 -> [_ w672]
          tunnel: w667 -> [_ w671]
          frame Default {
          }
          frame "/" {
            n453 = call <vilib>:"NT Update Persistence.vi"("Persistence"=w671, "Name"=w672) -> ()  [unwired: 9 in, 1 out]
          }
        }
      }
    }
  }
  n454 = while {
    tunnel: w64 -> [w674]
    i -> [w677]
    stop <- FALSE stop-if-true
    n455 = Wait (ms)(milliseconds to wait=u32 100) -> ()  [unwired: 1 out]
    n456 = case shown="\"Stop\", Default" "Rec Mode" {
      tunnel: w677 -> [_ _ w692]
      tunnel: [u32 2829099 ("Base Color") u32 11141120 ("Target Color") w681] -> w673
      frame "Stop", Default {
        # "Reset the color, extra updates don't cost much"
      }
      frame "Record" {
      }
      frame "Playback" {
        # "Playback"
        n457 = Quotient & Remainder(x=w692, y=u32 50 ("milliseconds to wait")) -> (x-y*floor(x/y)=w688:u32)  [unwired: 1 out]
        n458 = Divide(x=w688, y=u32 50 ("milliseconds to wait")) -> (x/y=w685:dbl)
        n459 = Multiply(x=6.283185307179586, y=w685) -> (x*y=w690:dbl)
        n460 = Sine(x=w690) -> (sin(x)=w689:dbl)
        n461 = Absolute Value(x=w689) -> (abs(x)=w682:dbl)
        n462 = call "Interpolate RGB Color.vi"("Proportion"=w682, "Target Color"=u32 30976, "Base Color"=u32 2829099) -> ("Result Color"=w681:u32)  [unwired: 8 in]
      }
    }
    n463 = property class="Pane"(reference=w674, "PaneColor"=w673) -> ()  [unwired: 1 in, 2 out]
  }
  n464 = disable-structure shown="Disabled" {
    frame Disabled {
      n465 = local write "Dashboard Tab"(T29."Basic" ("Dashboard Tab")) -> ()
    }
    frame Enabled {
    }
  }
  n466 = property on="On/Off" class="Bool (strict)"("Visible"=w35) -> ()  [unwired: 2 in, 2 out]
  n467 = property on="Motor" class="Clust (strict)"("Visible"=w35) -> ()  [unwired: 2 in, 2 out]
  n468 = property on="Progress" class="Clust (strict)"("Visible"=w35) -> ()  [unwired: 2 in, 2 out]
  n469 = property on="Test Ring" class="Ring (strict)"("Visible"=w35) -> ()  [unwired: 2 in, 2 out]
  n470 = property on="Rev/Fwd" class="Clust (strict)"("Visible"=w35) -> ()  [unwired: 2 in, 2 out]
  n471 = while {
    tunnel: u16 1741 ("timeout ms (25000)") -> [w695]
    stop <- FALSE stop-if-true
    n472 = TCP Create Listener(10:w695) -> (0:w694:errorcluster, 3:w696:refnum<k5>)  [unwired: 4 in, 1 out]
    n473 = case shown="Error" w694 {
      selector: w694 -> [w698 _]
      tunnel: w696 -> [w699 _]
      frame No Error {
        n474 = while {
          tunnel: w699 -> [w702]
          tunnel: w698 -> [w701]
          stop <- FALSE stop-if-true
          n475 = TCP Wait On Listener(8:w701, 11:w702) -> (0:w703:errorcluster, 4:w704:refnum<k5>)  [unwired: 2 in, 3 out]
          n476 = local write "TCP"(w704) -> ()
          n477 = case shown="No Error" w703 {
            frame No Error {
            }
            frame Error {
              n478 = Wait (ms)(milliseconds to wait=u32 1000) -> ()  [unwired: 1 out]
            }
          }
        }
      }
      frame Error {
        n479 = Wait (ms)(milliseconds to wait=u32 1000) -> ()  [unwired: 1 out]
      }
    }
  }
  n480 = local write "Command Selection"(u16 0 ("milliseconds to wait")) -> ()
  n481 = local write "Command Params"(string[][] [] ("Command Params")) -> ()
  n482 = global write "WPI_DashboardLogging Global.vi" "Recording"(w58) -> ()
  n483 = local write "Rec Mode"(w58) -> ()
  n484 = call <vilib>:"NT Write String.vi"("String"="Select Auto", "Name"="Auto Selector") -> ()  [unwired: 9 in, 1 out]
